vi "IRISS V2 Thorlabs.vi"() -> ()   [LabVIEW 2016]
uses:
  <vilib>/Analysis/Matrix/Datatypes/RealMatrix.ctl
  <vilib>/Math Plots/3D Math Plots/3D Scatter/3D Scatter XCtrl/3D Scatter.xctl
  Subsystems/Global Variables.vi
  <vilib>/Utility/file.llb/Read Delimited Spreadsheet (DBL).vi
  <vilib>/FPGAPlugInAG/PXI-7833R/niLvFpga_Open_PXI-7833R.vi
  <vilib>/Utility/error.llb/Error Cluster From Error Code.vi
  <vilib>/rvi/errors/niLvFpgaAdjustHostInterfaceError.vi
  <vilib>/Math Plots/3D Math Plots/3D Scatter/3D Scatter Datatype/Public/Plot Helper (Vector).vi
  Library/mjglib/var_OCTzHomeDir.vi
  <vilib>/FPGAPlugInAG/PXI-7833R/niLvFpga_Reset_PXI-7833R.vi
  <vilib>/FPGAPlugInAG/PXI-7833R/niLvFpga_Close_PXI-7833R.vi
  <vilib>/rvi/interface/nirviOpenFPGA/nirviOpenFPGA.xnode
  FPGA Bitfiles/PhantomControlPI_FPGATarget_QuadCtr2_E2412E44.lvbitx
  IRISS_FPGA_IO.vi
  <vilib>/rvi/interface/nirviReadWriteControl/nirviReadWriteControl.xnode
  <vilib>/Math Plots/3D Math Plots/3D Plot/3D Plot Datatype/3D Plot Datatype.lvclass
  <vilib>/rvi/interface/nirviMethod/nirviMethod.xnode
  <vilib>/rvi/interface/nirviCloseFPGA/nirviCloseFPGA.xnode
  <vilib>/Analysis/Matrix/NI_Matrix.lvlib
  Functions/EyeRobotDLL.dll
  Library/KevinLibraryAll/labview2011/kevLib2011.lvlib
  <vilib>/Math Plots/3D Math Plots/3D Scatter/3D Scatter Datatype/3D Scatter Datatype.lvclass
  NiFpgaLv.dll
panel:
  in  "Calib Params?":bool
  in  "Incision":bool caption="To M/S"
  out "Trajectory Cluster":T1
  in  "OCT Z PID Gains":cluster{"Kp":dbl, "Kd":dbl, "Ki":dbl}={"Kp"=0.0003, "Kd"=0.0001, "Ki"=0.01}
  out "deltaRoll":sgl
  out "deltaXYZ":sgl[](array[numeric])
  out "Online Eye Model":T2
  in  "To Regulation":bool
  out "Eye Model Cluster":T4={"X Grid"=[], "Y Grid"=[], "Za_true Surf"=[], "Iris Center"=[], "Zp_true Surf"=[], "Pinv"=[[1.0, 0.0], [0.0, 1.0]], "za_true"=5.0, "za_work"=1.0, "zp_work"=-1.0, "zp_true"=-5.0}
  out "Update Mdl & Traj":bool=TRUE
  in  "Initialize":bool caption="To M/S"
  in  "IRISS GUI":T5(tab)
  in  "U/S Power [%]":sgl min=0 max=100 step=10
  in  "Vac Cmd [mmHg]":sgl min=0 max=600 step=50
  in  "Red Round Box":u32(colorbox)=16711690
  in  "Blue Round Box":u32(colorbox)=16860
  in  "Black Round Box":u32(colorbox)
  out "Vacuum Force [mmHg]  2":i32 caption="[mmHg]"
  in  "IV Height [mmHg]":dbl=30.0 min=0.0 max=90.0 step=10.0
  in  "Irrigation":bool
  in  "Reroute Hold [sec]":dbl=10.0 caption="Hold [sec]"
  out "Next Speed":dbl=0.8 format="%#.2gx"
  out "Current Speed":dbl=0.2 format="%#_2gx"
  out "Next Depth":dbl=40.0 format="%#_g%%"
  out "Current Depth":dbl=20.0 format="%#_6g%%"
  in  "Depth Offset":dbl min=-30.0 max=70.0 step=5.0 format="%#_g%%"
  in  "Refractive Index":dbl=1.35
  in  "PO No-Fly":dbl=5.0 step=0.1 format="%#.2g"
  out "PO Cruising":dbl=5.0 format="%#.2g"
  in  "Iris Center":dbl=5.0 step=0.1 format="%#.2g"
  in  "AN Cruising":dbl=5.0 step=0.1 format="%#.2g"
  in  "AN No-Fly":dbl=5.0 step=0.1 format="%#.2g"
  in  "Iris XY Scaling":dbl[](array[numeric])=[1.0, 1.0] caption="Iris Scaling" min=0.5 max=2.0 step=0.05
  in  "Iris XY Center":dbl[](array[numeric])=[0.0, 5.0] caption="Iris Center" min=-5.0 max=5.0 step=0.25
  out "Asgn Pt Out of Bound":bool caption="Assign Pt OOB"
  out "Emergency alarm":bool
  out "Remote sender engaged":bool
  out "State changing":bool
  out "Current Run No.":u8
  out "No. of Runs":i32=5
  out "Tip out Posit":dbl[](array[numeric]) caption="Position [mm]" format="%#.3f"
  out "Tip cmd Posit":dbl[](array[numeric]) caption="Command [mm]" format="%#.3f"
  out "State Flag Array":bool[](array[boolean])
  in  "Speed Override":u16=3
  out "Timer":i32 format="%<%M:%S>t"
  in  "Assign Point [mm]":dbl[](array[numeric])=[0.0, -7.0, -6.0]
  in  "Go to Assign Pt":bool
  out "Irrigation Engaged?":bool caption="Irrigation Engaged"
  out "Robot XYZ":refnum<class "3D Plot Datatype.lvclass">[](xcontrol)
  in  "Offset":dbl[](array[numeric])
  in  "Radial Scale":dbl=0.5
  in  "Pattern":T6(ring)=enum."Centered"
  in  "Stop-and-Go":bool
  in  "SCAN_NO":string
  in  "Gen Traj":bool
  out "Trajectory OOB":bool
  out "Current System State":T7(ring)
  in  "Current Surgical Stage":T8(ring)
  in  "Tracking Mode":u16(ring) items=["Joint Mode", "XYZ Mode"]
  in  "Stage Z [mm]":dbl=100.0 min=-120.0 max=120.0 step=0.5
  in  "Stage Y [mm]":dbl=70.0 min=-120.0 max=100.0 step=0.5
  in  "Gripper":dbl
  in  "OCT Cmd Z [mm]":dbl min=-25.0 max=14.0 step=0.5
  out "Joint Out":dbl[](array[numeric])
  out "Robot Status Array":bool[](array[boolean])
  in  "L1 [deg]":dbl=-40.0
  in  "L2 [deg]":dbl=15.0
  in  "L3 [mm]":dbl=-5.0 step=0.1
  out "Status 2":bool[](array[boolean])
  in  "L4 [deg]":dbl=-10.0 step=0.1
  in  "Home":bool
  out "OCT Z out [mm]":dbl caption="OCT Out Z [mm]" format="%#.4f"
  in  "Tool Type":i32=6
  in  "Tool Offset [mm]":dbl=-50.68
  out "Grasp out":dbl format="%#.4g"
  in  "OCTz Home Dir":bool
  in  "Remote Control Source":u16(ring) caption="Remote Source" items=["None", "Surgical Console", "Joystick", "Rigid Joystick", "Zeiss PC", "MJG C++ Teleoperation", "A-Scan", "Free Joystick 2023", "Zeiss PC 2023", "MSR Zeiss Teleoperation"]
  in  "Reset Joystick":bool caption="Encoder Reset"
  out "Send Count":u64
  out "Receive Count":u64
  out "Arm ID Ind":i32
  out "Status":bool
  in  "Stage X [mm]":dbl=30.0 min=-120.0 max=120.0 step=0.5
  out "XYZ Stage out":dbl[](array[numeric])
  out "XYZ Stage cmd":dbl[](array[numeric])
  out "DH Params":cluster{"d_DH":dbl[][], "ty":dbl[][]}
  in  "Use Online Scan":bool
  in  "Process VSCAN":bool
  in  "Restart":bool
  out "Generation Error":errorcluster
  out "Model Created":bool
  in  "Eye No":i16=1 min=1 step=1
  in  "Reroute Transit Vacf":dbl=100.0
  in  "Z Rot Axis":dbl=1.0
  in  "Z Dist Thld":dbl[](array[numeric])=[3.0, 5.0] caption="Z Distance Threshould"
  in  "Vac Extremum":dbl[](array[numeric])=[68.0, 68.0] caption="Vacuum Extremum"
  in  "Max Limit [mmHg]":dbl=600.0 min=0.0 max=600.0 step=100.0
  out "Value [mmHg]":i8
  in  "Save Data":bool
  out "File Exists":bool
  out "File Path":path
  out "Elaspsed Time [s]":sgl
  in  "Data No":i16=1 min=1 step=1
  in  "Total Time":i16=90 min=1 step=1
  in  "Min PC Gap":dbl=0.1 caption="Min PC Gap [mm]" min=0.0 max=10.0 step=0.1 format="%#.3g"
  in  "Min AC Gap":dbl=0.1 caption="Min AC Gap [mm]" min=0.0 max=10.0 step=0.1 format="%#.3g"
  out "Scaling":dbl[](array[numeric])=[1.0, 1.0, 1.0] caption="S" min=0.5 max=1.5 step=0.05 format="%#_3g"
  in  "Joint Limits":dbl[][](array[numeric])=[[-68.0, -4.0], [-26.0, 52.0], [-40.0, 23.0], [-180.0, 180.0]] format="%#.3g"
  out "First Trk Pt":dbl[](array[numeric]) format="%#.3g"
  out "Error(s) Out on Program End":errorcluster
  out "L4 Waveform Graph":dbl[](graph)
  out "L3 Waveform Graph":dbl[](graph)
  out "L2 Waveform Graph":dbl[](graph)
  out "L1 Waveform Graph":dbl[](graph)
  in  "Aiming Pt":dbl[](array[numeric])=[-40.0, 11.0, 2.0, 0.0] format="%#.3g"
  in  "Engage Pt":dbl[](array[numeric])=[-40.0, 11.0, 2.0, 0.0] format="%#.3g"
  in  "Rotation":dbl[](array[numeric])=[0.0, 0.0, 0.0] caption="R [deg]" min=-15.0 max=15.0 step=0.5 format="%#_3g"
  out "Translation":dbl[](array[numeric]) caption="T [mm]" min=-3.0 max=3.0 step=0.1 format="%#_3g"
  in  "Inc Ctrl":dbl[](array[numeric])=[0.1, 0.05, 0.05] caption="Increment Control"
  in  "Depth Ctrl Array\n(% Thickness)":dbl[](array[numeric])=[40.0, 60.0, 80.0] min=10.0 max=90.0 step=5.0 format="%#_g%%"
  out "Stage command":dbl[](array[numeric])
  in  "Vscan path":path=path "D:/IRISSoft LV2016 beta/Host Demo/ThorlabsData/Eye1/VSCAN_0002.raw"
  in  "size_xyz_mm":dbl[](array[numeric])=[16.0, 16.0, 9.4, 1.0]
  in  "size_xyz":dbl[](array[numeric])=[400.0, 400.0, 1024.0, 1.0]
  in  "Confirm":bool
  in  "Image index":i32=200
  out "O":dbl[](array[numeric])
  out "New TOI":dbl[][](array[numeric])
  out "Original TOI":dbl[][](array[numeric])
  in  "Load Traj":bool caption="To M/S"
  in  "MS/Auto":bool
  in  "Retract":bool caption="To M/S"
  in  "Stop Accurus":bool caption="To M/S"
  in  "L3 Go Home":bool caption="To M/S"
  in  "Track":bool caption="To M/S"
  in  "Insert":bool caption="To M/S"
  in  "Program Stop":bool
  # "M/S\n \nAuto"
  # "Tool Tip Location"
  # "Tracking Planning"
  # "RCM"
  # "X\nY\nZ"
  # "X\nY\nZ"
  # "Tool"
  # "Trajectory"
  # "System Progress"
  # "Assign Point Rerouting"
  # "Trajectory Generation"
  # "X\nY\nZ"
  # "X Offset"
  # "Y Offset"
  # "Homing finished"
  # "Z Offset"
  # "M/S initialization finished"
  # "Tool Cruising Boundaries"
  # "XY-plane"
  # "Trajecoty loading finished"
  # "Aiming finished"
  # "Tool engaged"
  # "Z-axis"
  # "Phaco Machine"
  # "Tracking initialization finished"
  # "In Tracking"
  # "Rerouting finished"
  # "X\nY"
  # "X\nY"
  # "In regulation"
  # "Robot Control"
  # "Homing"
  # "Joint Definition"
  # "Arm"
  # "Tool"
  # "Stage"
  # "Robot Status"
  # "Joint M/S Cmd"
  # "HARDWARE_NOT_PRESENT"
  # "HARDWARE_NOT_FOUND_ALL_DRIVES"
  # "HARDWARE_SENSOR_FAULT"
  # "NOT_RUNNING"
  # "COMMUNICATION_ERROR"
  # "KINEMATICS_NO_SOLUTION"
  # "OCT Control"
  # "KINEMATICS_INSERTION_LENGTH_TOO_SMALL"
  # "COMMAND_BEYOND_JOINT_RANGE"
  # "COMMAND_TOO_LARGE"
  # "Eye Model Creation"
  # "Irrigation and Aspiration"
  # "IOP Control"
  # "Data Saving"
  # "Irrigation"
  # "Aspiration"
  # "ACh"
  # "Vitreous"
  # "Rotation & Vacuum Force Scheduling"
  # "Joint Motion & Control"
  # "Space Deform Parameters"
  # "Depth Ctrl"
  # "S"
  # "R"
  # "[deg]"
  # "T"
  # "[mm]"
  # "First Track Point"
  # "AC & PC Gap"
  # "X1"
  # "[mm]"
  # "Y"
  # "[mm]"
  # "Z"
  # "[mm]"
  # "L4"
  # "[deg]"
  # "Joint Limits"
  # "Error Message"
  # "Incision"
  # "Min."
  # "Max."
  # "L1"
  # "[deg]"
  # "L1"
  # "L2"
  # "L2"
  # "[deg]"
  # "L3"
  # "[mm]"
  # "L3"
  # "L4"
  # "[deg]"
  # "L4"
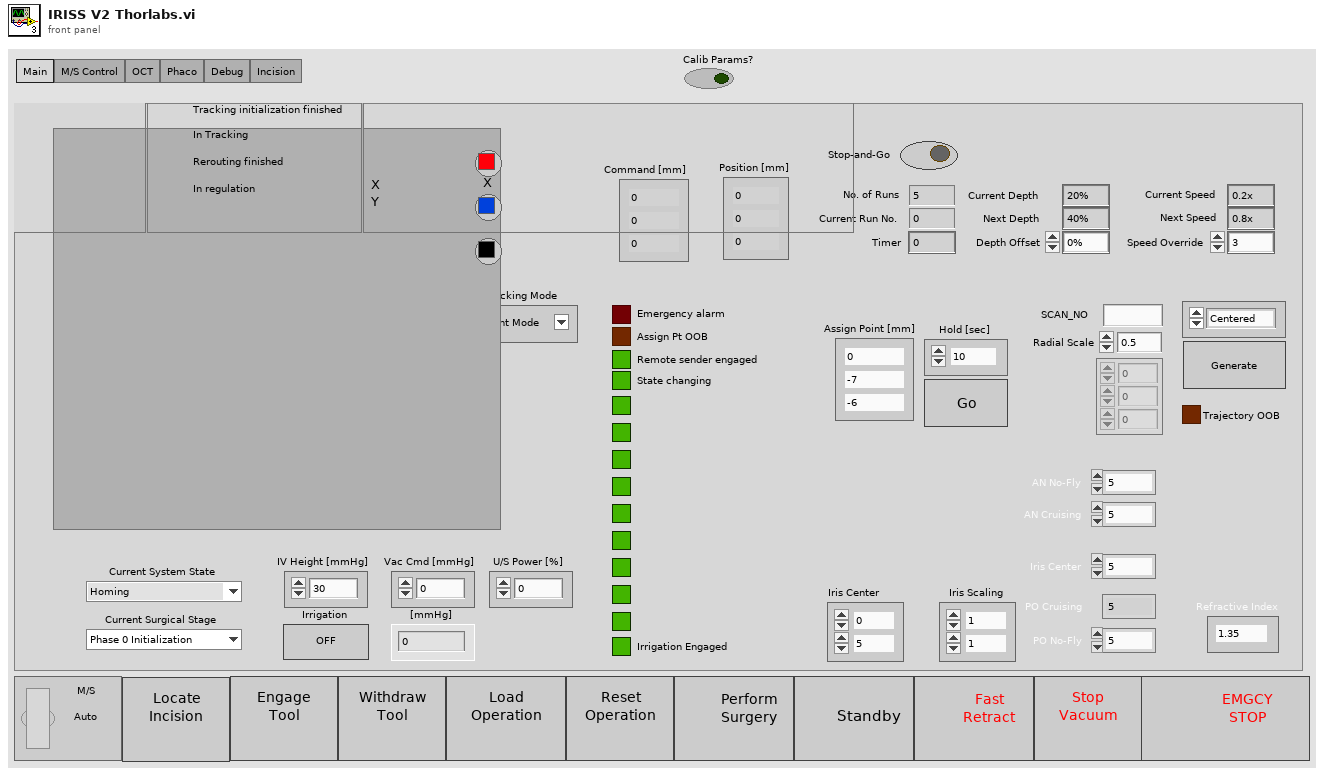
[diagram p1: front panel]
types:
  T1 = cluster{"Traj Px Array":dbl[], "Traj Py Array":dbl[], "Traj Pz Array":dbl[], "Speed Array":dbl[], "Depth Array":dbl[], "Traj Joint1 Array":dbl[], "Traj Joint2 Array":dbl[], "Traj Joint3 Array":dbl[], "Traj Joint4 Array":dbl[], "Traj Joint5 Array":dbl[]}
  T2 = cluster{"za_true":dbl, "za_work":dbl, "zi":dbl, "zp_work":dbl, "zp_true":dbl, "Iris XY Center":dbl[], "Iris XY Scaling":dbl[]}
  T3 = typedef "NI_Matrix.lvlib/RealMatrix.ctl" = dbl[][]
  T4 = cluster{"X Grid":dbl[], "Y Grid":dbl[], "Za_true Surf":dbl[][], "Iris Center":dbl[], "Zp_true Surf":dbl[][], "Pinv":T3, "za_true":dbl, "za_work":dbl, "zp_work":dbl, "zp_true":dbl}
  T5 = enum32{"Main", "M/S Control", "OCT", "Phaco", "Debug", "Incision"}
  T6 = enum16{"Entry Site", "Centered", "Insertion", "Extraction", "Reverse Entry Site", "Reverse Centered"}
  T7 = enum16{"Homing", "M/S Initialization", "M/S Operation", "Aiming", "Engaging", "Trajectory Loading", "Tracking Initialization", "Tracking", "Rerouting", "Regulation"}
  T8 = enum16{"Phase 0 Initialization", "Phase 1 Phaco", "Phase 2 Lens Removal", "Phase 3 IOL Injection"}
  T9 = enum8{"Enabled", "Disabled", "Disabled and Grayed Out"}
  T10 = cluster{"za_true_0":dbl, "za_work_0":dbl, "zp_work_0":dbl, "zp_true_0":dbl, "IrisCenter_0":dbl[]}
  T11 = cluster{"X Grid":dbl[], "Y Grid":dbl[], "Za_true Surf":dbl[][], "Iris Center":dbl[], "Zp_true Surf":dbl[][], "Real Matrix":T3, "za_true":dbl, "za_work":dbl, "zp_work":dbl, "zp_true":dbl}
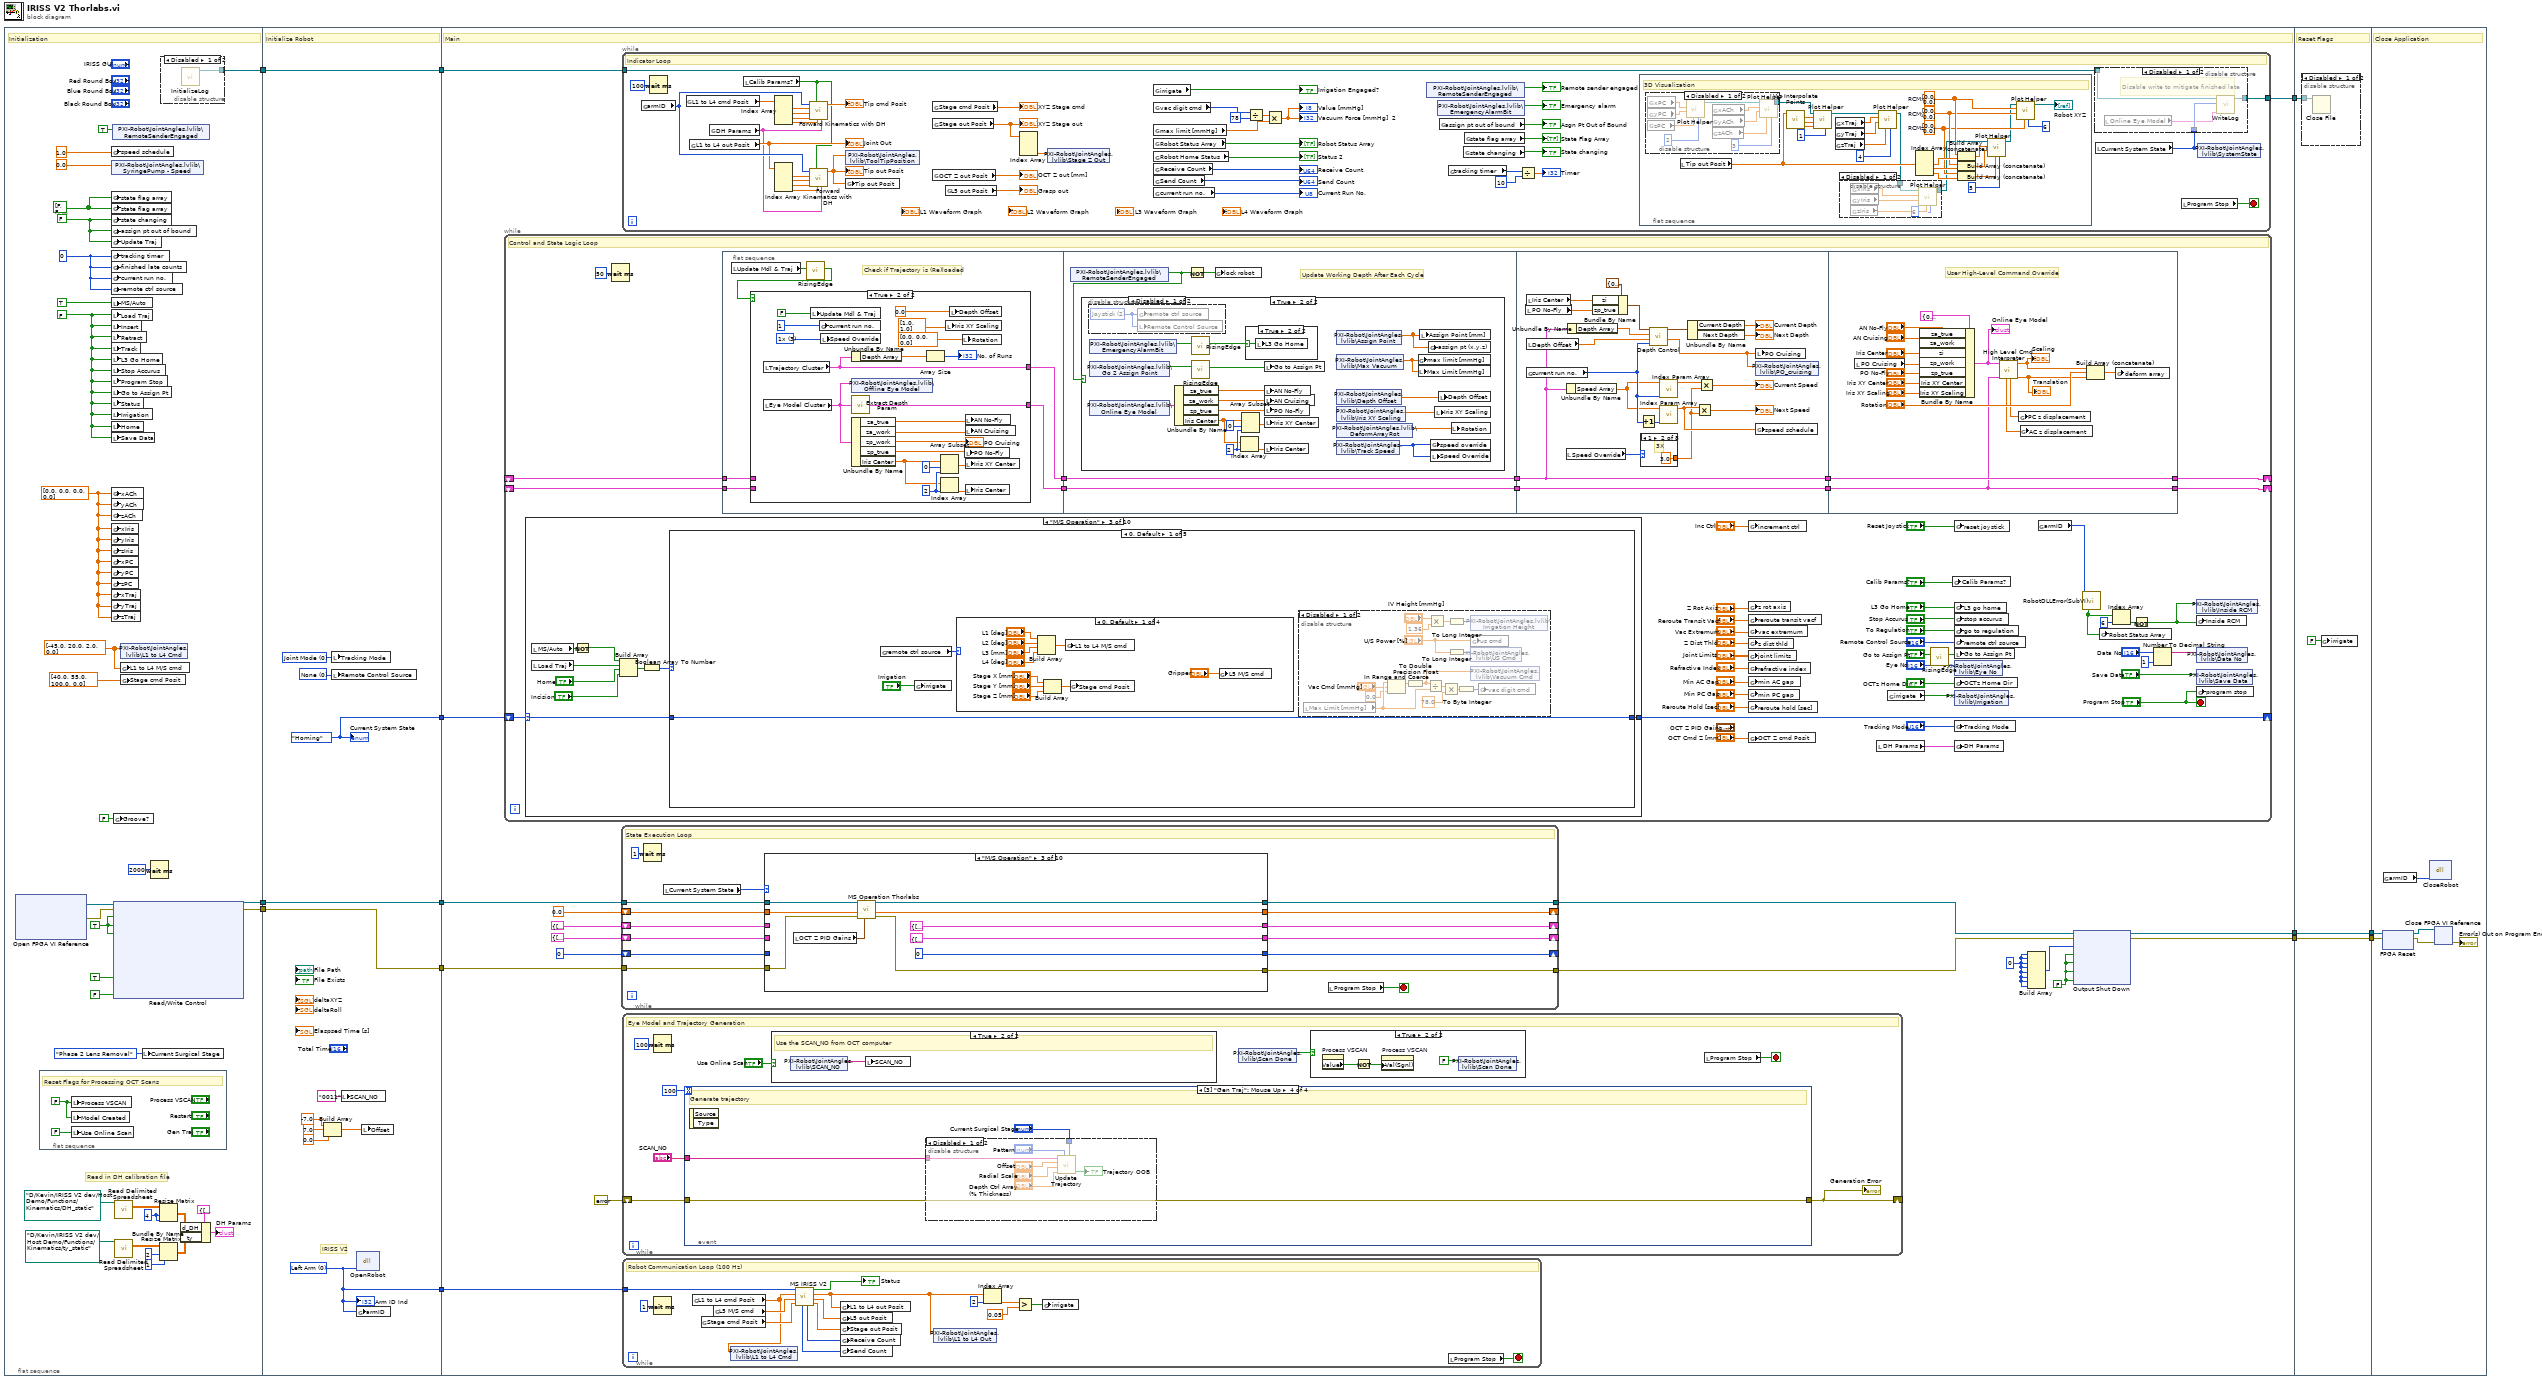
[diagram p0: block diagram]
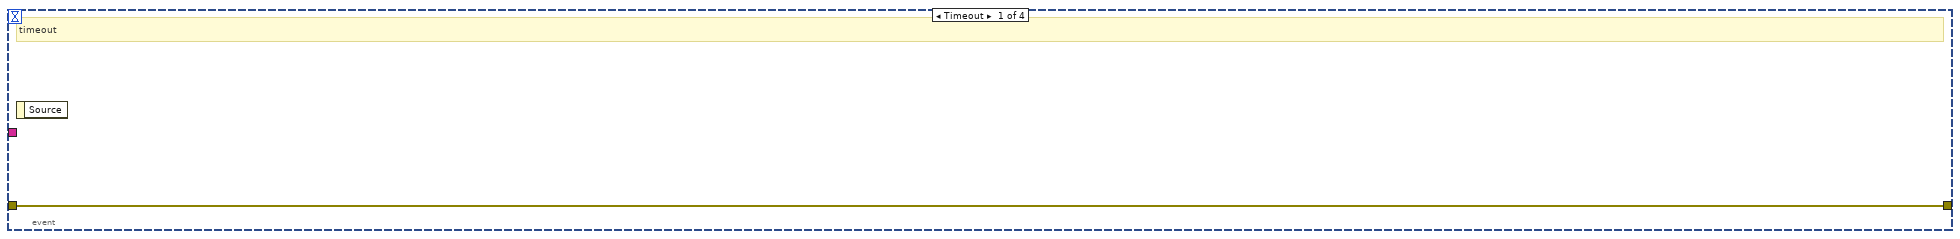
[diagram p5: hidden frame]
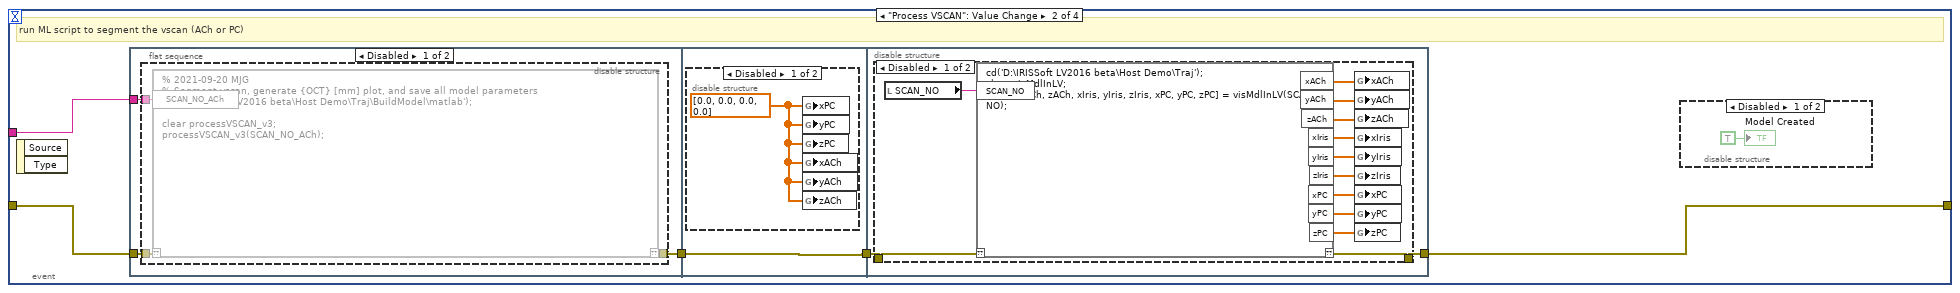
[diagram p6: hidden frame]
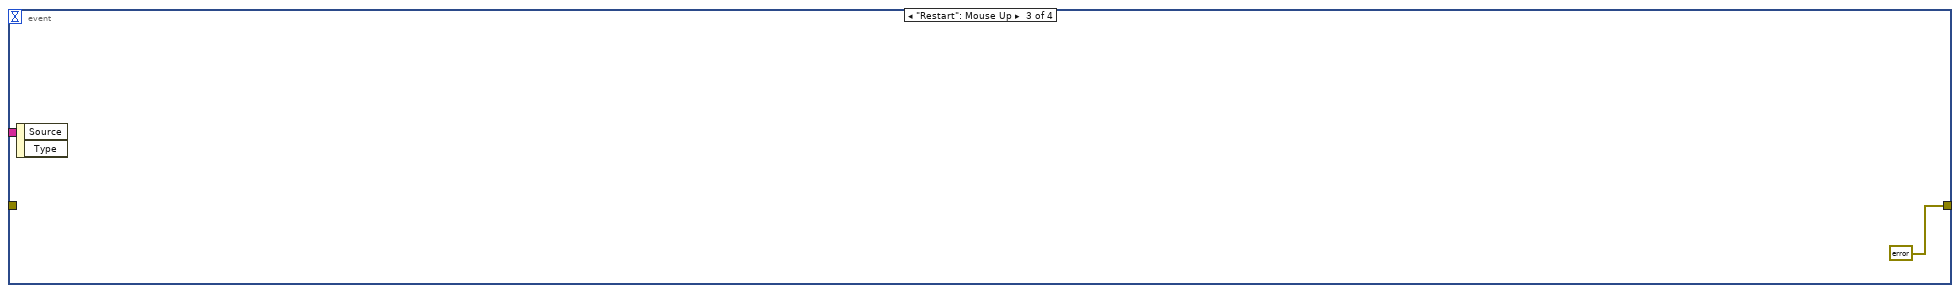
[diagram p11: hidden frame]
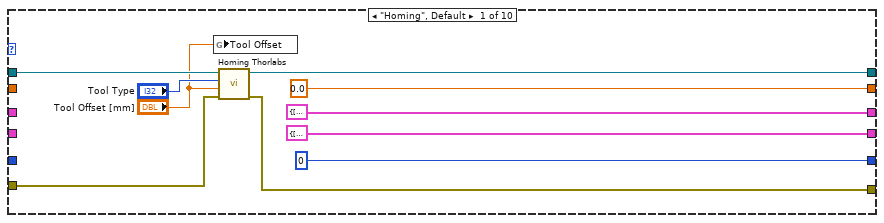
[diagram p13: hidden frame]
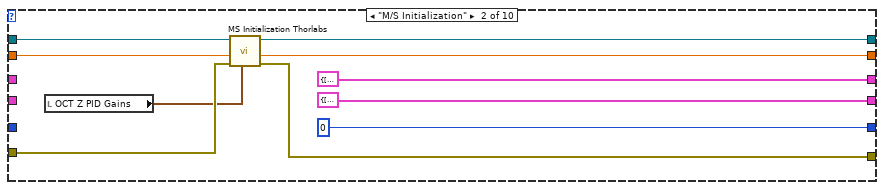
[diagram p14: hidden frame]
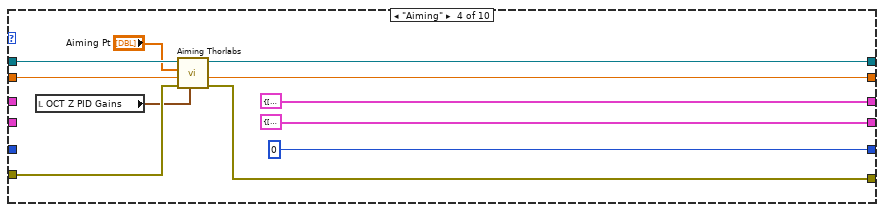
[diagram p15: hidden frame]
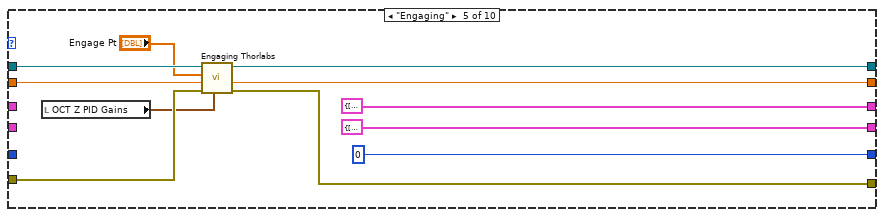
[diagram p16: hidden frame]
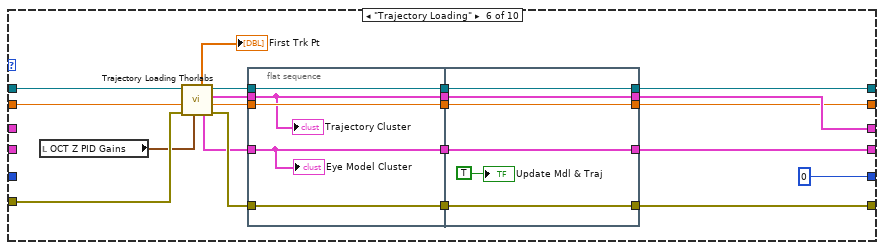
[diagram p17: hidden frame]
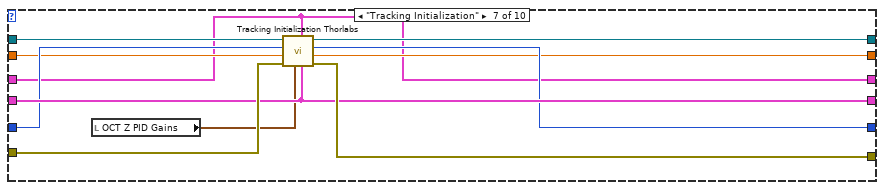
[diagram p18: hidden frame]
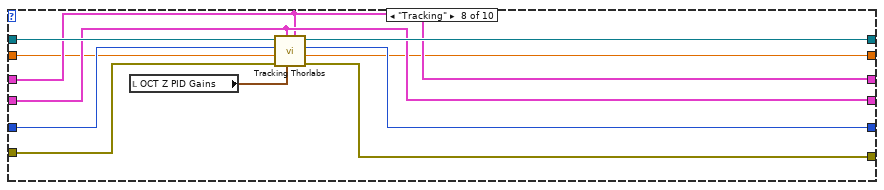
[diagram p19: hidden frame]
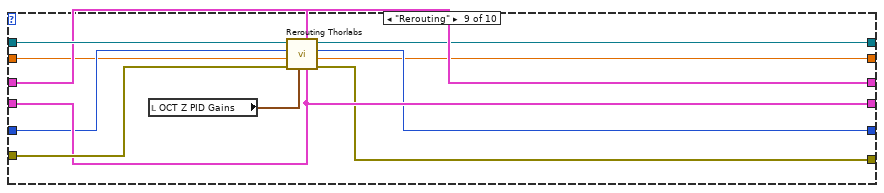
[diagram p20: hidden frame]
diagram:
  n1 = flat-sequence {
    tunnel: [w45] -> w5
    tunnel: [w37] -> w3
    tunnel: [w36] -> w2
    tunnel: [w59] -> w8
    tunnel: [w60] -> w7
    tunnel: [w58] -> w6
    tunnel: w5 -> [w61]
    tunnel: [w61] -> w4
    tunnel: w3 -> [w60]
    tunnel: w2 -> [w59]
    tunnel: [w51] -> w1
    tunnel: w8 -> [w76]
    tunnel: w7 -> [w73]
    tunnel: w6 -> [w79]
    tunnel: [w74] -> w13
    tunnel: [w75] -> w12
    tunnel: w4 -> [w78]
    tunnel: [w77] -> w11
    tunnel: w1 -> [w64]
    tunnel: w13 -> [w862]
    tunnel: w12 -> [w863]
    tunnel: w11 -> [w864]
    tunnel: [w863] -> w10
    tunnel: [w862] -> w9
    tunnel: w10 -> [w871]
    tunnel: w9 -> [w870]
    frame #0 {
      w22 = 4 ("number of rows")
      w38 = TRUE ("Conn0/DIO13 Button 2")
      w34 = dbl[] [0.0, 0.0, 0.0, 0.0] ("First Trk Pt 2")
      w29 = dbl[] [-45.0, 20.0, 2.0, 0.0] ("First Trk Pt 2")
      w33 = 0 ("finished late counts")
      w44 = bool[] [FALSE, FALSE, FALSE, FALSE, FALSE, FALSE, FALSE, FALSE, FALSE] ("state flag array")
      w42 = FALSE ("state changing")
      w35 = FALSE ("program stop")
      # "Read in DH calibration file"
      # "Initialization"
      n2 = xnode "Open FPGA VI Reference"() -> ("FPGA VI Reference Out"=w32:refnum<k20>, "error out"=w31:errorcluster)  [unwired: 2 in]
      n3 = flat-sequence {
        frame #0 {
          w47 = FALSE ("ACh Processed")
          # "Reset Flags for Processing OCT Scans"
          n4 = local write "Process VSCAN"(w47) -> ()
          n5 = local write "Model Created"(w47) -> ()
          n6 = local write "Use Online Scan"(FALSE ("Use Online Scan")) -> ()
        }
      }
      n7 = global write "Global Variables.vi" "speed schedule"(1.0 ("speed schedule")) -> ()
      n8 = shared-variable "PXI-Robot\\JointAngles.lvlib\\SyringePump - Speed"(0.0 ("SyringePump - Speed")) -> ()  [unwired: 1 in, 1 out]
      n9 = global write "Global Variables.vi" "state flag array"(w44) -> ()
      n10 = global write "Global Variables.vi" "state flag array"(w44) -> ()
      n11 = global write "Global Variables.vi" "state changing"(w42) -> ()
      n12 = global write "Global Variables.vi" "assign pt out of bound"(w42) -> ()
      n13 = global write "Global Variables.vi" "Update Traj"(w42) -> ()
      n14 = global write "Global Variables.vi" "tracking timer"(w33) -> ()
      n15 = global write "Global Variables.vi" "finished late counts"(w33) -> ()
      n16 = global write "Global Variables.vi" "current run no."(w33) -> ()
      n17 = global write "Global Variables.vi" "remote ctrl source"(w33) -> ()
      n18 = local write "MS/Auto"(TRUE ("MS/Auto")) -> ()
      n19 = local write "Load Traj"(w35) -> ()
      n20 = local write "Insert"(w35) -> ()
      n21 = local write "Retract"(w35) -> ()
      n22 = local write "Track"(w35) -> ()
      n23 = local write "L3 Go Home"(w35) -> ()
      n24 = local write "Stop Accurus"(w35) -> ()
      n25 = local write "Program Stop"(w35) -> ()
      n26 = local write "Go to Assign Pt"(w35) -> ()
      n27 = local write "Status"(w35) -> ()
      n28 = local write "Irrigation"(w35) -> ()
      n29 = local write "Home"(w35) -> ()
      n30 = local write "Save Data"(w35) -> ()
      n31 = global write "Global Variables.vi" "xACh"(w34) -> ()
      n32 = global write "Global Variables.vi" "yACh"(w34) -> ()
      n33 = global write "Global Variables.vi" "zACh"(w34) -> ()
      n34 = global write "Global Variables.vi" "xIris"(w34) -> ()
      n35 = global write "Global Variables.vi" "yIris"(w34) -> ()
      n36 = global write "Global Variables.vi" "zIris"(w34) -> ()
      n37 = global write "Global Variables.vi" "xPC"(w34) -> ()
      n38 = global write "Global Variables.vi" "yPC"(w34) -> ()
      n39 = global write "Global Variables.vi" "zPC"(w34) -> ()
      n40 = global write "Global Variables.vi" "xTraj"(w34) -> ()
      n41 = global write "Global Variables.vi" "yTraj"(w34) -> ()
      n42 = global write "Global Variables.vi" "zTraj"(w34) -> ()
      n43 = shared-variable "PXI-Robot\\JointAngles.lvlib\\RemoteSenderEngaged"(TRUE ("RemoteSenderEngaged")) -> ()  [unwired: 1 in, 1 out]
      n44 = global write "Global Variables.vi" "Groove?"(FALSE ("Groove?")) -> ()
      n45 = xnode "Read/Write Control"("FPGA VI Reference In"=w32, "error in"=w31, "Conn0/DIO12 Button 1"=w38, "Conn0/DIO13 Button 2"=w38, "Conn0/DIO15 Button 4"=w38, "Reset 14"=TRUE, "Hydration On/Off (Connector2/DIO28)"=FALSE) -> ("FPGA VI Reference Out"=w37:refnum<k20>, "error out"=w36:errorcluster)  [unwired: 3 in, 2 out]
      n46 = call-poly <vilib>:"Read Delimited Spreadsheet.vi"("file path (dialog if empty)"=path "D:/Kevin/IRISS V2 dev/Host Demo/Functions/Kinematics/DH_static" ("file path (use dialog)")) -> ("all rows"=w23:dbl[][])  [unwired: 9 in, 5 out]
      n47 = call-poly <vilib>:"Read Delimited Spreadsheet.vi"("file path (dialog if empty)"=path "D:/Kevin/IRISS V2 dev/Host Demo/Functions/Kinematics/ty_static" ("file path (use dialog)")) -> ("all rows"=w21:dbl[][])  [unwired: 9 in, 5 out]
      n48 = shared-variable "PXI-Robot\\JointAngles.lvlib\\L1 to L4 Cmd"(w29) -> ()  [unwired: 1 in, 1 out]
      n49 = global write "Global Variables.vi" "L1 to L4 M/S cmd"(w29) -> ()
      n50 = global write "Global Variables.vi" "Stage cmd Posit"(dbl[] [40.0, 55.0, 100.0, 0.0] ("First Trk Pt 2")) -> ()
      n51 = local write "Current Surgical Stage"(T8."Phase 2 Lens Removal" ("Current Surgical Stage")) -> ()
      n52 = Wait (ms)(milliseconds to wait=u32 2000) -> ()  [unwired: 1 out]
      n53 = Resize Matrix(1:w22, 2:w22, 4:w23) -> (0:w17:dbl[][])
      n54 = Resize Matrix(1:1 ("number of columns"), 2:2 ("number of rows"), 4:w21) -> (0:w16:dbl[][])
      n55 = disable-structure shown="Disabled" {
        disable-tunnel: [w49 _] -> w45
        frame Disabled {
          n56 = call "InitializeLog.vi"() -> ("Byte Stream File out"=w49:refnum<file>)  [unwired: 11 in]
        }
        frame Enabled {
        }
      }
      n57 = Bundle By Name(cluster=cluster{"d_DH":dbl[][], "ty":dbl[][]} {"d_DH"=[[0.0, -0.04858099004841317, 1.1971672750675049, 0.0], [0.0, -1.576475511297109, 0.0, 0.0], [-0.3552491783526254, 0.0, -1.1064589410656984, 0.2058446720735121], [-1.0573457532495087, 1.0278049025155533, 0.011917110633363169, -0.004023577880993236]], "ty"=[[0.04320445582455471], [0.011728642746432275]]} ("input cluster"), "d_DH"=w17, "ty"=w16) -> (→"DH Params":cluster{"d_DH":dbl[][], "ty":dbl[][]})
    }
    frame #1 {
      w50 = u16 0 items=["Joint Mode", "XYZ Mode"] ("Tracking Mode")
      w57 = u16 0 items=["None", "Surgical Console", "Joystick", "MJG Teleoperation", "MJG C++ Teleoperation"] ("Remote Control Source 2")
      w58 = T7."Homing" ("Current State")
      w51 = 0 items=["Left Arm", "Right Arm"] ("Left or Right Arm")
      # "IRISS V2"
      # "Initialize Robot"
      n58 = Build Array(-7.0 ("element"), 7.0 ("element"), 0.0 ("element")) -> (w56:dbl[])
      n59 = local write "Tracking Mode"(w50) -> ()
      n60 = local write "Remote Control Source"(w57) -> ()
      n61 = local write "SCAN_NO"("0011" ("SCAN_NO")) -> ()
      n62 = dll-call lib="D:/Kevin/IRISS V2 dev/Host Demo/Functions/EyeRobotDLL.dll" fn="OpenRobot" label="Open"("id"=w51) -> ()  [unwired: 5 in, 2 out]
      n63 = global write "Global Variables.vi" "armID"(w51) -> ()
      n64 = local write "Offset"(w56) -> ()
      "Arm ID Ind" <- w51
      "Current System State" <- w58
    }
    frame #2 {
      w67 = FALSE
      w65 = i16 0 ("element")
      # "Main"
      n65 = while {
        shift-right: [w418] -> _
        shift-left: w79 -> [w419]
        shift-right: [w415] -> _
        shift-left: _ -> [w413]
        shift-right: [w414] -> _
        shift-left: _ -> [w412]
        stop <- "Program Stop" stop-if-true
        # "Control and State Logic Loop"
        n66 = case shown="\"M/S Operation\"" w419 {
          selector: w419 -> [w533 w540 w567 w653 w673 w699 w708 w739 w783 w811]
          tunnel: [w532 w541 w566 w652 w674 w700 w709 w740 w784 w812] -> w418
          frame "Homing", Default {
            # "State Diagram"
            n67 = global read "Global Variables.vi" "state flag array"() -> (w534:bool[])
            n68 = Index Array(array=w534, index=0) -> (element=w531:bool)
            n69 = case shown="False" w531 {
              tunnel: [w536 w538] -> w532
              tunnel: w533 -> [w536 _]
              frame False {
                # "homing in process"
              }
              frame True {
                w538 = T7."M/S Initialization" ("Current State")
                # "finish homing"
                n70 = global write "Global Variables.vi" "state changing"(TRUE ("state changing")) -> ()
                n71 = global write "Global Variables.vi" "Enforce Homing"(FALSE ("Enforce Homing")) -> ()
                n72 = local write "Current System State"(w538) -> ()
              }
            }
          }
          frame "M/S Initialization" {
            n73 = global read "Global Variables.vi" "state flag array"() -> (w543:bool[])
            n74 = Index Array(array=w543, index=1) -> (element=w542:bool)
            n75 = case shown="False" w542 {
              tunnel: [w554 w556] -> w541
              tunnel: w540 -> [w554 _]
              frame False {
                n76 = global read "Global Variables.vi" "Stage cmd Posit"() -> (w548:dbl[])
                n77 = property on="MS/Auto" class="Bool (strict)"("DisabledEnum"=T9."Disabled and Grayed Out" ("Disabled")) -> ()  [unwired: 2 in, 2 out]
                n78 = Index Array(array=w548) -> (element #1=w546:dbl, element #2=w547:dbl, element #3=w545:dbl)  [unwired: 3 in]
                n79 = global read "Global Variables.vi" "L1 to L4 M/S cmd"() -> (w553:dbl[])
                n80 = local write "Stage X [mm]"(w546) -> ()
                n81 = local write "Stage Y [mm]"(w547) -> ()
                n82 = local write "Stage Z [mm]"(w545) -> ()
                n83 = Index Array(array=w553) -> (element #1=w552:dbl, element #2=w551:dbl, element #3=w550:dbl, element #4=w549:dbl)  [unwired: 4 in]
                n84 = local write "L1 [deg]"(w552) -> ()
                n85 = local write "L2 [deg]"(w551) -> ()
                n86 = local write "L3 [mm]"(w550) -> ()
                n87 = local write "L4 [deg]"(w549) -> ()
              }
              frame True {
                w556 = T7."M/S Operation" ("Current State")
                n88 = global write "Global Variables.vi" "state changing"(TRUE ("state changing")) -> ()
                n89 = property on="MS/Auto" class="Bool (strict)"("DisabledEnum"=T9."Enabled" ("Disabled")) -> ()  [unwired: 2 in, 2 out]
                n90 = local write "Current System State"(w556) -> ()
              }
            }
          }
          frame "M/S Operation" {
            n91 = local read "MS/Auto"() -> (w565:bool)
            n92 = local read "Load Traj"() -> (w563:bool)
            n93 = Not(x=w565) -> (.not. x?=w564:bool)
            n94 = Build Array(w564, w563, "Home", "Incision") -> (w562:bool[])
            n95 = Boolean Array To Number(Boolean array=w562) -> (number=w561:u32)
            n96 = case shown="0, Default" w561 {
              tunnel: w567 -> [w570 _ w610 _ w619]
              tunnel: [w570 w606 w611 w618 w619] -> w566
              frame 0, Default {
                n97 = global read "Global Variables.vi" "remote ctrl source"() -> (w569:u16)
                n98 = global write "Global Variables.vi" "irrigate"("Irrigation") -> ()
                n99 = case shown="0, Default" w569 {
                  frame 0, Default {
                    n100 = Build Array("L1 [deg]", "L2 [deg]", "L3 [mm]", "L4 [deg]") -> (w586:dbl[])
                    n101 = Build Array("Stage X [mm]", "Stage Y [mm]", "Stage Z [mm]") -> (w591:dbl[])
                    n102 = global write "Global Variables.vi" "L1 to L4 M/S cmd"(w586) -> ()
                    n103 = global write "Global Variables.vi" "Stage cmd Posit"(w591) -> ()
                    n104 = global write "Global Variables.vi" "L5 M/S cmd"("Gripper") -> ()
                  }
                  frame 1 {
                    n105 = local read "OCT Cmd Z [mm]"() -> (w596:dbl)
                    n106 = global write "Global Variables.vi" "OCT Z cmd Posit"(w596) -> ()
                  }
                  frame 2 {
                    n107 = global read "Global Variables.vi" "Stage cmd Posit"() -> (w605:dbl[])
                    n108 = Index Array(array=w605) -> (element #1=w604:dbl, element #2=w603:dbl, element #3=w602:dbl)  [unwired: 3 in]
                    n109 = local write "Stage X [mm]"(w604) -> ()
                    n110 = local write "Stage Y [mm]"(w603) -> ()
                    n111 = local write "Stage Z [mm]"(w602) -> ()
                    n112 = global read "Global Variables.vi" "L1 to L4 cmd Posit"() -> (w597:dbl[])
                    n113 = Index Array(array=w597) -> (element #1=w600:dbl, element #2=w599:dbl, element #3=w598:dbl, element #4=w601:dbl)  [unwired: 4 in]
                    n114 = local write "L1 [deg]"(w600) -> ()
                    n115 = local write "L2 [deg]"(w599) -> ()
                    n116 = local write "L3 [mm]"(w598) -> ()
                    n117 = local write "L4 [deg]"(w601) -> ()
                  }
                  frame 3 {
                  }
                }
                n118 = disable-structure shown="Disabled" {
                  frame Disabled {
                    n119 = local read "Max Limit [mmHg]"() -> (w577:dbl)
                    n120 = In Range and Coerce(upper limit=w577, x="Vac Cmd [mmHg]", lower limit=0.0) -> (coerced(x)=w578:dbl)  [unwired: 1 out]
                    n121 = To Double Precision Float(number=w578) -> (double precision float=w579:dbl)
                    n122 = Divide(x=w579, y=w577) -> (x/y=w572:dbl)
                    n123 = Multiply(x="IV Height [mmHg]", y=1.36) -> (x*y=w583:dbl)
                    n124 = Multiply(x=w572, y=78.0) -> (x*y=w574:dbl)
                    n125 = To Long Integer(number=w583) -> (32bit integer=w584:i32)
                    n126 = To Long Integer(number="U/S Power [%]") -> (32bit integer=w580:i32)
                    n127 = To Byte Integer(number=w574) -> (8bit integer=w571:i8)
                    n128 = shared-variable "PXI-Robot\\JointAngles.lvlib\\Irrigation Height"(w584) -> ()  [unwired: 1 in, 1 out]
                    n129 = global write "Global Variables.vi" "us cmd"("U/S Power [%]") -> ()
                    n130 = shared-variable "PXI-Robot\\JointAngles.lvlib\\US Cmd"(w580) -> ()  [unwired: 1 in, 1 out]
                    n131 = shared-variable "PXI-Robot\\JointAngles.lvlib\\Vacuum Cmd"(w579) -> ()  [unwired: 1 in, 1 out]
                    n132 = global write "Global Variables.vi" "vac digit cmd"(w571) -> ()
                  }
                  frame Enabled {
                  }
                }
              }
              frame 1 {
                w606 = T7."Aiming" ("Current State")
                n133 = global write "Global Variables.vi" "state changing"(TRUE ("state changing")) -> ()
                n134 = local write "Current System State"(w606) -> ()
                n135 = property on="MS/Auto" class="Bool (strict)"("DisabledEnum"=T9."Disabled and Grayed Out" ("Disabled")) -> ()  [unwired: 2 in, 2 out]
              }
              frame 2 {
                n136 = global read "Global Variables.vi" "Inside RCM"() -> (w609:bool)
                n137 = case shown="True" w609 {
                  tunnel: [w612 w613] -> w611
                  tunnel: w610 -> [w612 _]
                  frame False {
                  }
                  frame True {
                    w613 = T7."Trajectory Loading" ("Current State")
                    w614 = FALSE ("MS/Auto")
                    n138 = global write "Global Variables.vi" "state changing"(TRUE ("state changing")) -> ()
                    n139 = local write "MS/Auto"(w614) -> ()
                    n140 = local write "Load Traj"(w614) -> ()
                    n141 = local write "Current System State"(w613) -> ()
                    n142 = property on="MS/Auto" class="Bool (strict)"("DisabledEnum"=T9."Disabled and Grayed Out" ("Disabled")) -> ()  [unwired: 2 in, 2 out]
                  }
                }
              }
              frame 4 {
                w618 = T7."Homing" ("Current State")
                w617 = TRUE ("state changing")
                n143 = global write "Global Variables.vi" "state changing"(w617) -> ()
                n144 = global write "Global Variables.vi" "Enforce Homing"(w617) -> ()
                n145 = local write "Current System State"(w618) -> ()
              }
              frame 8 {
                n146 = flat-sequence {
                  frame #0 {
                    n147 = while {
                      shift-right: [w626] -> _
                      shift-left: 0 -> [w627]
                      shift-right: [w624] -> _
                      shift-left: 1 -> [w625]
                      stop <- "Confirm" stop-if-true
                      n148 = script code="if index>400\n  index_ = 400;\nelseif index<=0\n  index_ = 1;\nelse\n  index_ = index;\nend"("index"="Image index") -> ("index_"=w626:dbl)  [unwired: 1 in, 1 out]
                      n149 = Wait (ms)(milliseconds to wait=u32 100) -> ()  [unwired: 1 out]
                      n150 = Not Equal?(x=w627, y=w626) -> (x != y?=w628:bool)
                      n151 = case shown="True" w628 {
                        tunnel: w626 -> [_ w637]
                        tunnel: w625 -> [w630 w635]
                        tunnel: [w630 w634] -> w624
                        frame False {
                        }
                        frame True {
                          n152 = Path To String(path="Vscan path") -> (string=w636:string)
                          n153 = script code="%size_xyz = [400 400 1024];\nsize_xyz = size_xyz(1:3);\nframe = 1;\n% showBscanImage(filename,frame,index,size_xyz,size_xyz_mm,first_time);\nif first_time\n  fid = fopen(filename);\n  % Read the intensity values (n x 1) vector (takes some time)\n  vscan = fread(fid, prod(size_xyz), 'float32');\n  vscan = reshape(vscan, flip(size_xyz));\n\n  % nicely scale the vscan\n  vscan = vscan2nice(vscan);\n  vscan = uint8(vscan);\nend\nif frame==0\n  new_size0 = [256 int32(256*size_xyz_mm(2)/size_xyz_mm(3))];\n  img0 = filplr(imresize(vscan(:,:,index),new_size0));\n  figure(1);imshow(img0);title(['Frame:0 Index:' num2str(index)]);\nelseif frame==1\n  new_size1 = [256 int32(256*size_xyz_mm(1)/size_xyz_mm(3))];\n  temp = vscan(:,index,:);\n  img1 = reshape(temp,[size(temp,1) size(temp,3)]);\n  img1 = fliplr(imresize(img1,new_size1));\n  figure(1);imshow(img1);title(['Frame:1 Index:' num2str(index)]);\nend\n\nfirst_time = 0;"("index"=w637, "size_xyz_mm"="size_xyz_mm", "size_xyz"="size_xyz", "filename"=w636, "first_time"=w635) -> ("first_time"=w634:dbl)  [unwired: 1 in, 1 out]
                        }
                      }
                      n154 = local write "Image index"(w626) -> ()
                    }
                  }
                  frame #1 {
                    n155 = local read "size_xyz_mm"() -> (w649:dbl[])
                    n156 = local read "Image index"() -> (w650:i32)
                    n157 = local read "Vscan path"() -> (w647:path)
                    n158 = local read "size_xyz"() -> (w648:dbl[])
                    n159 = Path To String(path=w647) -> (string=w646:string)
                    n160 = script code="%size_xyz_mm = [16 16 9.4];\n%size_xyz = [400 400 1024];\nsize_xyz = size_xyz(1:3);\nframe = 1;\n%INJECTloc_OCT=IOLSEG3(filename,frame,index,size_xyz,size_xyz_mm);\n\nif frame==0\n  image = fliplr(vscan(:,:,index));\n  size_xz_mm = [size_xyz_mm(2) size_xyz_mm(3)];\n  px2mm = size_xz_mm./[size_xyz(2) size_xyz(3)]; \nelseif frame==1\n  temp = vscan(:,index,:);\n  image = fliplr(reshape(temp,[size(temp,1) size(temp,3)]));\n  size_xz_mm = [size_xyz_mm(1) size_xyz_mm(3)];\n  px2mm = size_xz_mm./[size_xyz(1) size_xyz(3)]; \nend\n%% Only to look at the center scan plan\nfigure(2); clf; \nimshow(image); hold on;\n    \n% Collect two user clicks of Injection location \n[input1, Zinput1] = ginput(1);\nplot(input1, Zinput1, 'rx', 'MarkerSize', 20, 'LineWidth', 3); \n[input2, Zinput2] = ginput(1); % Collect two user clicks \nplot(input2, Zinput2, 'rx', 'MarkerSize', 20, 'LineWidth', 3); \n    \nYinput1 = size_xyz(2) - input1; \nYinput2 = size_xyz(2) - input2;\n    \nINJECTloc_px = [Yinput1, Zinput1; ... \n        Yinput2, Zinput2]; % [px] \nINJECTloc_px_mid=[(INJECTloc_px(1,1)+INJECTloc_px(2,1))/2,(INJECTloc_px(2,1)+INJECTloc_px(2,2))/2];\nclose(2); % close figure\n    \n% Convert these two locations from pixels to {OCT} frame  \nxloc_OCT = index/400*size_xz_mm(1); % B-scan is halfway through the image\nINJECTloc_OCT = [xloc_OCT*ones(1,1), INJECTloc_px_mid(1,1)*px2mm(1),  INJECTloc_px_mid(1,2)*px2mm(2)];\n\nincision_pt = [INJECTloc_OCT(1:3),1]';\nTOI_file= 'D:\\IRISSoft LV2016 beta\\Host Demo\\TOI_static'\nfid_TOI = fopen(TOI_file,'r');\nTOI=fscanf(fid_TOI,'%f');\nTOI= reshape(TOI, [4 4])';\nfclose(fid_TOI);\n\nO = inv(TOI)*incision_pt;\n%init_X = 40;init_Y = 55;init_Z = 100;\n%time_to_go = norm(O(1:3))/.5;\n%traj = [linspace(0,O(1),1000*time_to_go);linspace(0,O(2),1000*time_to_go);linspace(0,O(3),1000*time_to_go)];\n%stage_X = linspace(init_X,init_X+O(1),1000*time_to_go);\n%stage_Y = linspace(init_Y,init_Y+O(2),1000*time_to_go);\n%stage_Z = linspace(init_Z,init_Z+O(3),1000*time_to_go);\n\nTOI2 = inv(TOI);TOI2(1:3,4) = TOI2(1:3,4)-O(1:3);\nTOI2 = inv(TOI2);\nO = O';\n\nTOI2_file= 'D:\\IRISSoft LV2016 beta\\Host Demo\\new_TOI.txt';\nfid_TOI2 = fopen(TOI2_file,'w');\nfmt = [repmat('%.10f ', 1, 4), '\\n'];\nfprintf(fid_TOI2, fmt, TOI2');\nfclose(fid_TOI2);"("index"=w650, "size_xyz_mm"=w649, "size_xyz"=w648, "filename"=w646) -> ("TOI"=→"Original TOI":dbl[][], "TOI2"=→"New TOI":dbl[][], "O"=w643:dbl[])  [unwired: 1 in, 1 out]
                    "O" <- w643
                    n161 = local read "XYZ Stage out"() -> (w642:dbl[])
                    n162 = Add(x=w643, y=w642) -> (x+y=w641:dbl[])
                    "Stage command" <- w641
                    n163 = Index Array(array=w641) -> (element #1=w640:dbl, element #2=w639:dbl, element #3=w638:dbl)  [unwired: 3 in]
                    n164 = local write "Stage X [mm]"(w640) -> ()
                    n165 = local write "Stage Y [mm]"(w639) -> ()
                    n166 = local write "Stage Z [mm]"(w638) -> ()
                  }
                  frame #2 {
                    n167 = local write "Incision"(FALSE) -> ()
                  }
                }
              }
            }
          }
          frame "Aiming" {
            n168 = global read "Global Variables.vi" "state flag array"() -> (w655:bool[])
            n169 = Index Array(array=w655, index=3) -> (element=w654:bool)
            n170 = case shown="True" w654 {
              tunnel: w653 -> [w657 w661]
              tunnel: [w657 w660] -> w652
              frame False {
              }
              frame True {
                n171 = property on="MS/Auto" class="Bool (strict)"("DisabledEnum"=T9."Enabled" ("Disabled")) -> ()  [unwired: 2 in, 2 out]
                n172 = Build Array("Insert", "MS/Auto") -> (w665:bool[])
                n173 = Boolean Array To Number(Boolean array=w665) -> (number=w662:u32)
                n174 = case shown="1" w662 {
                  tunnel: w661 -> [w666 _ _]
                  tunnel: [w666 w667 w671] -> w660
                  frame 0, Default {
                  }
                  frame 1 {
                    w667 = T7."Engaging" ("Current State")
                    n175 = global write "Global Variables.vi" "state changing"(TRUE ("state changing")) -> ()
                    n176 = local write "Insert"(FALSE ("Enter")) -> ()
                    n177 = property on="MS/Auto" class="Bool (strict)"("DisabledEnum"=T9."Disabled and Grayed Out" ("Disabled")) -> ()  [unwired: 2 in, 2 out]
                    n178 = local write "Current System State"(w667) -> ()
                  }
                  frame 2 {
                    w671 = T7."M/S Initialization" ("Current State")
                    n179 = global write "Global Variables.vi" "state changing"(TRUE ("state changing")) -> ()
                    n180 = local write "Current System State"(w671) -> ()
                  }
                }
                n181 = local read "OCT Cmd Z [mm]"() -> (w658:dbl)
                n182 = global write "Global Variables.vi" "OCT Z cmd Posit"(w658) -> ()
              }
            }
          }
          frame "Engaging" {
            n183 = global read "Global Variables.vi" "state flag array"() -> (w676:bool[])
            n184 = Index Array(array=w676, index=4) -> (element=w675:bool)
            n185 = case shown="True" w675 {
              tunnel: [w679 w686] -> w674
              tunnel: w673 -> [w680 w687]
              frame False {
                n186 = local read "Retract"() -> (w678:bool)
                n187 = case shown="False" w678 {
                  tunnel: [w681 w682] -> w679
                  tunnel: w680 -> [w681 _]
                  frame False {
                  }
                  frame True {
                    w682 = T7."Aiming" ("Current State")
                    n188 = global write "Global Variables.vi" "state changing"(TRUE ("state changing")) -> ()
                    n189 = local write "Retract"(FALSE ("Retract")) -> ()
                    n190 = local write "Current System State"(w682) -> ()
                  }
                }
              }
              frame True {
                n191 = Build Array("Load Traj", "Retract") -> (w690:bool[])
                n192 = Boolean Array To Number(Boolean array=w690) -> (number=w688:u32)
                n193 = case shown="2" w688 {
                  tunnel: w687 -> [w691 _ _]
                  tunnel: [w691 w692 w695] -> w686
                  frame 0, Default {
                  }
                  frame 1 {
                    w692 = T7."Trajectory Loading" ("Current State")
                    n194 = global write "Global Variables.vi" "state changing"(TRUE ("state changing")) -> ()
                    n195 = local write "Load Traj"(FALSE ("Load Traj")) -> ()
                    n196 = local write "Current System State"(w692) -> ()
                  }
                  frame 2 {
                    w695 = T7."Aiming" ("Current State")
                    n197 = global write "Global Variables.vi" "state changing"(TRUE ("state changing")) -> ()
                    n198 = local write "Retract"(FALSE ("Load Traj")) -> ()
                    n199 = local write "Current System State"(w695) -> ()
                  }
                }
              }
            }
          }
          frame "Trajectory Loading" {
            n200 = global read "Global Variables.vi" "state flag array"() -> (w702:bool[])
            n201 = global write "Global Variables.vi" "irrigate"(TRUE ("irrigate")) -> ()
            n202 = Index Array(array=w702, index=2) -> (element=w701:bool)
            n203 = case shown="False" w701 {
              tunnel: [w704 w705] -> w700
              tunnel: w699 -> [w704 _]
              frame False {
              }
              frame True {
                w705 = T7."Tracking Initialization" ("Current State")
                n204 = global write "Global Variables.vi" "state changing"(TRUE ("state changing")) -> ()
                n205 = local write "Current System State"(w705) -> ()
              }
            }
          }
          frame "Tracking Initialization" {
            n206 = global read "Global Variables.vi" "state flag array"() -> (w711:bool[])
            n207 = Index Array(array=w711, index=5) -> (element=w710:bool)
            n208 = case shown="True" w710 {
              tunnel: [w713 w720] -> w709
              tunnel: w708 -> [w713 w719]
              frame False {
              }
              frame True {
                n209 = local read "Load Traj"() -> (w721:bool)
                n210 = local read "Retract"() -> (w715:bool)
                n211 = local read "To Regulation"() -> (w714:bool)
                n212 = Or(x="Initialize", y=w715) -> (x .or. y?=w717:bool)
                n213 = Build Array("Track", w721, w717, w714) -> (w723:bool[])
                n214 = Boolean Array To Number(Boolean array=w723) -> (number=w722:u32)
                n215 = case shown="1" w722 {
                  tunnel: [w724 w725 w728 w731 w734] -> w720
                  tunnel: w719 -> [w724 _ _ _ _]
                  frame 0, Default {
                  }
                  frame 1 {
                    w725 = T7."Tracking" ("Current State")
                    n216 = global write "Global Variables.vi" "state changing"(TRUE ("state changing")) -> ()
                    n217 = local write "Track"(FALSE ("Track")) -> ()
                    n218 = local write "Current System State"(w725) -> ()
                  }
                  frame 2 {
                    w728 = T7."Trajectory Loading" ("Current State")
                    n219 = global write "Global Variables.vi" "state changing"(TRUE ("state changing")) -> ()
                    n220 = local write "Load Traj"(FALSE ("Load Traj")) -> ()
                    n221 = local write "Current System State"(w728) -> ()
                  }
                  frame 4 {
                    w731 = T7."Engaging" ("Current State")
                    n222 = global write "Global Variables.vi" "state changing"(TRUE ("state changing")) -> ()
                    n223 = local write "Initialize"(FALSE ("Load Traj")) -> ()
                    n224 = local write "Current System State"(w731) -> ()
                  }
                  frame 8 {
                    w734 = T7."Tracking" ("Current State")
                    w735 = FALSE  # Reset
                    n225 = global write "Global Variables.vi" "state changing"(TRUE ("state changing")) -> ()
                    n226 = local write "Track"(FALSE ("Track")) -> ()
                    n227 = local write "Current System State"(w734) -> ()
                    n228 = local write "To Regulation"(w735) -> ()
                  }
                }
              }
            }
            n229 = global write "Global Variables.vi" "irrigate"(TRUE ("irrigate")) -> ()
          }
          frame "Tracking" {
            n230 = global read "Global Variables.vi" "state flag array"() -> (w742:bool[])
            n231 = global write "Global Variables.vi" "irrigate"(TRUE ("irrigate")) -> ()
            n232 = Index Array(array=w742, index=6) -> (element=w741:bool)
            n233 = case shown="True" w741 {
              tunnel: [w744 w765] -> w740
              tunnel: w739 -> [w744 w764]
              frame False {
              }
              frame True {
                (unwired) 90 ("y")
                # "2022-08-09 Kevin\nPhaco one groove at a time"
                n234 = global read "Global Variables.vi" "Groove?"() -> (w745:bool)
                n235 = local read "Initialize"() -> (w761:bool)
                n236 = local read "Retract"() -> (w758:bool)
                n237 = local read "Go to Assign Pt"() -> (w759:bool)
                n238 = local read "To Regulation"() -> (w760:bool)
                n239 = local read "Timer"() -> (w757:i32)
                n240 = local read "Total Time"() -> (w749:i16)
                n241 = global write "Global Variables.vi" "irrigate"(TRUE ("irrigate")) -> ()
                n242 = Quotient & Remainder(x=w757, y=w749) -> (x-y*floor(x/y)=w756:i32, floor(x/y)=w752:i32)
                n243 = Equal To 0?(x=w756) -> (x = 0?=w755:bool)
                n244 = Not Equal To 0?(x=w752) -> (x != 0?=w751:bool)
                n245 = call "RisingEdge.vi"("Signal In"=w755) -> ("Rising Edge"=w754:bool)  [unwired: 10 in]
                n246 = feedback #1() -> (w747:bool)  [unwired: 1 in]
                n247 = feedback-in #1(w745) -> ()
                n248 = Compound Arithmetic op=AND(w754, w751, "Stop-and-Go") -> ()  [unwired: 1 out]
                n249 = Not Equal?(x=w745, y=w747) -> (x != y?=w746:bool)
                n250 = Build Array(w761, w758, w759, w760, FALSE ("element"), w746) -> (w763:bool[])
                n251 = Boolean Array To Number(Boolean array=w763) -> (number=w762:u32)
                n252 = case shown="32" w762 {
                  tunnel: [w766 w767 w770 w773 w776 w779 w781] -> w765
                  tunnel: w764 -> [w766 _ _ _ _ _ _]
                  frame 0, Default {
                  }
                  frame 1 {
                    w767 = T7."Engaging" ("Current State")
                    n253 = global write "Global Variables.vi" "state changing"(TRUE ("state changing")) -> ()
                    n254 = local write "Initialize"(FALSE ("Load Traj")) -> ()
                    n255 = local write "Current System State"(w767) -> ()
                  }
                  frame 2 {
                    w770 = T7."Aiming" ("Current State")
                    n256 = global write "Global Variables.vi" "state changing"(TRUE ("state changing")) -> ()
                    n257 = local write "Retract"(FALSE ("Load Traj")) -> ()
                    n258 = local write "Current System State"(w770) -> ()
                  }
                  frame 4 {
                    w773 = T7."Rerouting" ("Current State")
                    n259 = global write "Global Variables.vi" "state changing"(TRUE ("state changing")) -> ()
                    n260 = local write "Go to Assign Pt"(FALSE ("Load Traj")) -> ()
                    n261 = local write "Current System State"(w773) -> ()
                  }
                  frame 8 {
                    w776 = T7."Regulation" ("Current State")
                    n262 = global write "Global Variables.vi" "state changing"(TRUE ("state changing")) -> ()
                    n263 = local write "Current System State"(w776) -> ()
                  }
                  frame 16 {
                    w779 = T7."Regulation" ("Current State")
                    w778 = TRUE ("state changing")
                    n264 = global write "Global Variables.vi" "state changing"(w778) -> ()
                    n265 = local write "To Regulation"(w778) -> ()
                    n266 = local write "Current System State"(w779) -> ()
                  }
                  frame 32 {
                    w781 = T7."Trajectory Loading" ("Current State")
                    n267 = global write "Global Variables.vi" "state changing"(TRUE ("state changing")) -> ()
                    n268 = local write "Current System State"(w781) -> ()
                  }
                }
              }
            }
          }
          frame "Rerouting" {
            n269 = global read "Global Variables.vi" "state flag array"() -> (w786:bool[])
            n270 = Index Array(array=w786, index=7) -> (element=w785:bool)
            n271 = case shown="True" w785 {
              tunnel: [w790 w804] -> w784
              tunnel: w783 -> [w789 _]
              frame False {
                n272 = shared-variable "PXI-Robot\\JointAngles.lvlib\\EmergencyAlarmBit"() -> (w796:bool)  [unwired: 1 in, 1 out]
                n273 = local read "Initialize"() -> (w795:bool)
                n274 = local read "Retract"() -> (w788:bool)
                n275 = local read "Go to Assign Pt"() -> (w792:bool)
                n276 = Compound Arithmetic op=OR(w796, w795, w788) -> (w793:bool)
                n277 = Build Array(w793, w792) -> (w794:bool[])
                n278 = Boolean Array To Number(Boolean array=w794) -> (number=w791:u32)
                n279 = case shown="2" w791 {
                  tunnel: w789 -> [w797 _ _]
                  tunnel: [w797 w798 w801] -> w790
                  frame 0, Default {
                  }
                  frame 1 {
                    w798 = T7."Engaging" ("Current State")
                    n280 = global write "Global Variables.vi" "state changing"(TRUE ("state changing")) -> ()
                    n281 = local write "Initialize"(FALSE ("Initialize")) -> ()
                    n282 = local write "Current System State"(w798) -> ()
                  }
                  frame 2 {
                    w801 = T7."Rerouting" ("Current State")
                    n283 = global write "Global Variables.vi" "state changing"(TRUE ("state changing")) -> ()
                    n284 = local write "Go to Assign Pt"(FALSE ("Initialize")) -> ()
                    n285 = local write "Current System State"(w801) -> ()
                  }
                }
              }
              frame True {
                n286 = local read "To Regulation"() -> (w805:bool)
                n287 = case shown="False" w805 {
                  tunnel: [T7."Tracking" ("Current State") T7."Regulation" ("Current State")] -> w804
                  frame False {
                    n288 = global write "Global Variables.vi" "state changing"(TRUE ("state changing")) -> ()
                  }
                  frame True {
                    n289 = global write "Global Variables.vi" "state changing"(TRUE ("state changing")) -> ()
                  }
                }
                n290 = local write "Current System State"(w804) -> ()
              }
            }
            n291 = global write "Global Variables.vi" "irrigate"(TRUE ("irrigate")) -> ()
          }
          frame "Regulation" {
            n292 = global read "Global Variables.vi" "state flag array"() -> (w814:bool[])
            n293 = global write "Global Variables.vi" "irrigate"(TRUE ("irrigate")) -> ()
            n294 = Index Array(array=w814, index=8) -> (element=w813:bool)
            n295 = case shown="True" w813 {
              tunnel: [w823 w835] -> w812
              tunnel: w811 -> [w822 w836]
              frame False {
                n296 = local read "Initialize"() -> (w821:bool)
                n297 = local read "Retract"() -> (w820:bool)
                n298 = local read "Go to Assign Pt"() -> (w816:bool)
                n299 = Or(x=w821, y=w820) -> (x .or. y?=w819:bool)
                n300 = Build Array(w819, w816) -> (w818:bool[])
                n301 = Boolean Array To Number(Boolean array=w818) -> (number=w817:u32)
                n302 = case shown="2" w817 {
                  tunnel: w822 -> [w824 _ _]
                  tunnel: [w824 w826 w829] -> w823
                  frame 0, Default {
                  }
                  frame 1 {
                    w825 = FALSE  # Reset
                    w826 = T7."Engaging" ("Current State")
                    n303 = global write "Global Variables.vi" "state changing"(TRUE ("state changing")) -> ()
                    n304 = local write "Initialize"(FALSE ("Load Traj")) -> ()
                    n305 = local write "Current System State"(w826) -> ()
                    n306 = local write "To Regulation"(w825) -> ()
                  }
                  frame 2 {
                    w829 = T7."Rerouting" ("Current State")
                    n307 = global write "Global Variables.vi" "state changing"(TRUE ("state changing")) -> ()
                    n308 = local write "Go to Assign Pt"(FALSE ("Initialize")) -> ()
                    n309 = local write "Current System State"(w829) -> ()
                  }
                }
              }
              frame True {
                n310 = local read "Load Traj"() -> (w838:bool)
                n311 = local read "Go to Assign Pt"() -> (w839:bool)
                n312 = local read "Initialize"() -> (w834:bool)
                n313 = local read "Retract"() -> (w832:bool)
                n314 = local read "Track"() -> (w833:bool)
                n315 = Build Array(w838, w839, w834, w832, w833) -> (w840:bool[])
                n316 = Boolean Array To Number(Boolean array=w840) -> (number=w837:u32)
                n317 = case shown="8" w837 {
                  tunnel: w836 -> [w841 _ _ _ _ _]
                  tunnel: [w841 w843 w846 w850 w854 w858] -> w835
                  frame 0, Default {
                  }
                  frame 1 {
                    w842 = FALSE  # Reset
                    w843 = T7."Trajectory Loading" ("Current State")
                    n318 = global write "Global Variables.vi" "state changing"(TRUE ("state changing")) -> ()
                    n319 = local write "Load Traj"(FALSE ("Load Traj")) -> ()
                    n320 = local write "Current System State"(w843) -> ()
                    n321 = local write "To Regulation"(w842) -> ()
                  }
                  frame 2 {
                    w846 = T7."Rerouting" ("Current State")
                    n322 = global write "Global Variables.vi" "state changing"(TRUE ("state changing")) -> ()
                    n323 = local write "Go to Assign Pt"(FALSE ("Load Traj")) -> ()
                    n324 = local write "Current System State"(w846) -> ()
                  }
                  frame 4 {
                    w849 = FALSE  # Reset
                    w850 = T7."Engaging" ("Current State")
                    n325 = global write "Global Variables.vi" "state changing"(TRUE ("state changing")) -> ()
                    n326 = local write "Initialize"(FALSE ("Load Traj")) -> ()
                    n327 = local write "To Regulation"(w849) -> ()
                    n328 = local write "Current System State"(w850) -> ()
                  }
                  frame 8 {
                    w853 = FALSE  # Reset
                    w854 = T7."Aiming" ("Current State")
                    n329 = global write "Global Variables.vi" "state changing"(TRUE ("state changing")) -> ()
                    n330 = local write "Retract"(FALSE ("Load Traj")) -> ()
                    n331 = local write "To Regulation"(w853) -> ()
                    n332 = local write "Current System State"(w854) -> ()
                  }
                  frame 16 {
                    w857 = FALSE  # Reset
                    w858 = T7."Tracking" ("Current State")
                    n333 = global write "Global Variables.vi" "state changing"(TRUE ("state changing")) -> ()
                    n334 = local write "Track"(FALSE ("Load Traj")) -> ()
                    n335 = local write "Current System State"(w858) -> ()
                    n336 = local write "To Regulation"(w857) -> ()
                  }
                }
              }
            }
          }
        }
        n337 = Wait (ms)(milliseconds to wait=u32 50) -> ()  [unwired: 1 out]
        n338 = flat-sequence {
          tunnel: [w432] -> w404
          tunnel: [w431] -> w403
          tunnel: w413 -> [w430]
          tunnel: w412 -> [w429]
          tunnel: w404 -> [w460]
          tunnel: w403 -> [w459]
          tunnel: [w460] -> w402
          tunnel: [w459] -> w401
          tunnel: w402 -> [w488]
          tunnel: [w488] -> w400
          tunnel: w401 -> [w505]
          tunnel: [w505] -> w399
          tunnel: w400 -> [w528]
          tunnel: w399 -> [w518]
          tunnel: [w518] -> w414
          tunnel: [w528] -> w415
          frame #0 {
            # "Check if Trajectory is (Re)loaded"
            n339 = local read "Update Mdl & Traj"() -> (w434:bool)
            n340 = call "RisingEdge.vi"("Signal In"=w434) -> ("Rising Edge"=w433:bool)  [unwired: 10 in]
            n341 = case shown="True" w433 {
              tunnel: [w435 w456] -> w431
              tunnel: [w436 w445] -> w432
              tunnel: w430 -> [w436 _]
              tunnel: w429 -> [w435 _]
              frame False {
                # "Use Nominal Model & Trajectory"
              }
              frame True {
                w438 = u16 3 items=["4x", "3x", "2x", "1x", "0.5x", "0.2x", "0.1x", "PAUSE"] ("Speed Override")
                w450 = 2 ("index")
                # "Update Trajectory and Model after \"Trajectory Loading\""
                n342 = local read "Trajectory Cluster"() -> (w445:T1)
                n343 = local read "Eye Model Cluster"() -> (w443:T4)
                n344 = local write "Update Mdl & Traj"(FALSE ("Update Model")) -> ()
                n345 = global write "Global Variables.vi" "current run no."(u8 1 ("current run no.")) -> ()
                n346 = local write "Speed Override"(w438) -> ()
                n347 = Unbundle By Name(w445) -> ("Depth Array"=w447:dbl[])
                n348 = shared-variable "PXI-Robot\\JointAngles.lvlib\\Offline Eye Model"(w443) -> ()  [unwired: 1 in, 1 out]
                n349 = call "Extract Depth Param.vi"("Eye Model Cluster"=w443) -> ("Nominal Model param"=w456:T10)
                n350 = Unbundle By Name(w443) -> ("za_true"=w455:dbl, "za_work"=w454:dbl, "zp_work"=→"PO Cruising":dbl, "zp_true"=w452:dbl, "Iris Center"=w449:dbl[])
                n351 = Array Size(array=w447) -> (size(s)=→"No. of Runs":i32)
                n352 = Index Array(array=w449, index=w450) -> (element=w453:dbl)
                n353 = Array Subset(array=w449, index=0, length=w450) -> (w448:dbl[])
                n354 = local write "Iris XY Scaling"(dbl[] [1.0, 1.0]) -> ()
                n355 = local write "Depth Offset"(0.0 ("Depth Offset")) -> ()
                n356 = local write "Rotation"(dbl[] [0.0, 0.0, 0.0]) -> ()
                n357 = local write "PO No-Fly"(w452) -> ()
                n358 = local write "AN No-Fly"(w455) -> ()
                n359 = local write "AN Cruising"(w454) -> ()
                n360 = local write "Iris XY Center"(w448) -> ()
                n361 = local write "Iris Center"(w453) -> ()
              }
            }
          }
          frame #1 {
            # "Update Working Depth After Each Cycle"
            n362 = shared-variable "PXI-Robot\\JointAngles.lvlib\\RemoteSenderEngaged"() -> (w457:bool)  [unwired: 1 in, 1 out]
            n363 = case shown="True" w457 {
              frame False {
                n364 = global write "Global Variables.vi" "assign pt (x,y,z)"("Assign Point [mm]") -> ()
                n365 = global write "Global Variables.vi" "max limit [mmHg]"("Max Limit [mmHg]") -> ()
                n366 = global write "Global Variables.vi" "speed override"("Speed Override") -> ()
              }
              frame True {
                w468 = 2 ("index")
                n367 = disable-structure shown="Disabled" {
                  frame Disabled {
                    w483 = u16 2 items=["None", "Surgical Console", "Joystick", "MJG Teleoperation", "MJG C++ Teleoperation"] ("Remote Control Source 2")
                    n368 = global write "Global Variables.vi" "remote ctrl source"(w483) -> ()
                    n369 = local write "Remote Control Source"(w483) -> ()
                  }
                  frame Enabled {
                  }
                }
                n370 = shared-variable "PXI-Robot\\JointAngles.lvlib\\EmergencyAlarmBit"() -> (w480:bool)  [unwired: 1 in, 1 out]
                n371 = shared-variable "PXI-Robot\\JointAngles.lvlib\\Go 2 Assign Point"() -> (w477:bool)  [unwired: 1 in, 1 out]
                n372 = shared-variable "PXI-Robot\\JointAngles.lvlib\\Online Eye Model"() -> (w473:T11)  [unwired: 1 in, 1 out]
                n373 = Unbundle By Name(w473) -> ("za_true"=w476:dbl, "za_work"=w475:dbl, "zp_true"=w474:dbl, "Iris Center"=w465:dbl[])
                n374 = call "RisingEdge.vi"("Signal In"=w480) -> ("Rising Edge"=w479:bool)  [unwired: 10 in]
                n375 = call "RisingEdge.vi"("Signal In"=w477) -> ("Rising Edge"=w478:bool)  [unwired: 10 in]
                n376 = Index Array(array=w465, index=w468) -> (element=w466:dbl)
                n377 = Array Subset(array=w465, index=0, length=w468) -> (w469:dbl[])
                n378 = case shown="True" w479 {
                  selector: w479 -> [_ w484]
                  frame False {
                  }
                  frame True {
                    n379 = local write "L3 Go Home"(w484) -> ()
                  }
                }
                n380 = local write "Go to Assign Pt"(w478) -> ()
                n381 = local write "AN No-Fly"(w476) -> ()
                n382 = local write "AN Cruising"(w475) -> ()
                n383 = local write "PO No-Fly"(w474) -> ()
                n384 = local write "Iris XY Center"(w469) -> ()
                n385 = local write "Iris Center"(w466) -> ()
                n386 = shared-variable "PXI-Robot\\JointAngles.lvlib\\Assign Point"() -> (w481:dbl[])  [unwired: 1 in, 1 out]
                n387 = shared-variable "PXI-Robot\\JointAngles.lvlib\\Max Vacuum"() -> (w464:dbl)  [unwired: 1 in, 1 out]
                n388 = shared-variable "PXI-Robot\\JointAngles.lvlib\\Depth Offset"() -> (w472:dbl)  [unwired: 1 in, 1 out]
                n389 = shared-variable "PXI-Robot\\JointAngles.lvlib\\Iris XY Scaling"() -> (w471:dbl[])  [unwired: 1 in, 1 out]
                n390 = shared-variable "PXI-Robot\\JointAngles.lvlib\\DeformArrayRot"() -> (w470:dbl[])  [unwired: 1 in, 1 out]
                n391 = shared-variable "PXI-Robot\\JointAngles.lvlib\\Track Speed"() -> (w482:u16)  [unwired: 1 in, 1 out]
                n392 = global write "Global Variables.vi" "max limit [mmHg]"(w464) -> ()
                n393 = local write "Max Limit [mmHg]"(w464) -> ()
                n394 = local write "Assign Point [mm]"(w481) -> ()
                n395 = global write "Global Variables.vi" "assign pt (x,y,z)"(w481) -> ()
                n396 = global write "Global Variables.vi" "speed override"(w482) -> ()
                n397 = local write "Speed Override"(w482) -> ()
                n398 = local write "Iris XY Scaling"(w471) -> ()
                n399 = local write "Depth Offset"(w472) -> ()
                n400 = local write "Rotation"(w470) -> ()
              }
            }
            n401 = Not(x=w457) -> (.not. x?=w458:bool)
            n402 = global write "Global Variables.vi" "lock robot"(w458) -> ()
          }
          frame #2 {
            n403 = local read "PO No-Fly"() -> (w499:dbl)
            n404 = local read "Iris Center"() -> (w500:dbl)
            n405 = local read "Depth Offset"() -> (w504:dbl)
            n406 = global read "Global Variables.vi" "current run no."() -> (w497:u8)
            n407 = local read "Speed Override"() -> (w494:u16)
            n408 = Unbundle By Name(w488) -> ("Speed Array"=w496:dbl[])
            n409 = Unbundle By Name(w488) -> ("Depth Array"=w495:dbl[])
            n410 = Bundle By Name(cluster=cluster{"zi":dbl, "zp_true":dbl} {"zi"=0.0, "zp_true"=-2.5} ("z Cluster"), "zi"=w500, "zp_true"=w499) -> (w486:cluster{"zi":dbl, "zp_true":dbl})
            n411 = Increment(x=w497) -> (x+1=w498:u8)
            n412 = case shown="1" w494 {
              tunnel: [4.0 ("y") 3.0 ("y") 2.0 ("y") 1.0 ("y") 0.5 ("y") 0.2 ("y") 0.1 ("y") 0.0 ("y")] -> w491
              frame 0 {
                # "4X"
              }
              frame 1 {
                # "3X"
              }
              frame 2 {
                # "2X"
              }
              frame 3, Default {
                # "1x"
              }
              frame 4 {
                # "0.5x"
              }
              frame 5 {
                # "0.2x"
              }
              frame 6 {
                # "0.1x"
              }
              frame 7 {
                # "Pause"
              }
            }
            n413 = call "Depth Control.vi"("Current Run No."=w497, "Depth Offset"=w504, "Depth Array"=w495, "z Cluster"=w486) -> ("zp_work"=w485:dbl, "Schedule Depth & Speed"=w503:cluster{"Next Depth":dbl, "Current Depth":dbl})  [unwired: 6 in]
            n414 = call "Index Param Array.vi"("Index"=w497, "Array Input"=w496) -> ("Index Output"=w492:dbl)  [unwired: 9 in]
            n415 = call "Index Param Array.vi"("Index"=w498, "Array Input"=w496) -> ("Index Output"=w493:dbl)  [unwired: 9 in]
            n416 = Unbundle By Name(w503) -> ("Current Depth"=→"Current Depth":dbl, "Next Depth"=→"Next Depth":dbl)
            n417 = Multiply(x=w493, y=w491) -> (x*y=→"Next Speed":dbl)
            n418 = Multiply(x=w492, y=w491) -> (x*y=→"Current Speed":dbl)
            n419 = local write "PO Cruising"(w485) -> ()
            n420 = shared-variable "PXI-Robot\\JointAngles.lvlib\\PO_cruising"(w485) -> ()  [unwired: 1 in, 1 out]
            n421 = global write "Global Variables.vi" "speed schedule"(w493) -> ()
          }
          frame #3 {
            # "User High-Level Command Override"
            n422 = local read "PO Cruising"() -> (w520:dbl)
            n423 = Bundle By Name(cluster=T2 {"za_true"=0.0, "za_work"=0.0, "zi"=0.0, "zp_work"=0.0, "zp_true"=0.0, "Iris XY Center"=[0.0, 5.0], "Iris XY Scaling"=[1.0, 1.0]} ("High Level cmd"), "za_true"="AN No-Fly", "za_work"="AN Cruising", "zi"="Iris Center", "zp_work"=w520, "zp_true"="PO No-Fly", "Iris XY Center"="Iris XY Center", "Iris XY Scaling"="Iris XY Scaling") -> (w519:T2)
            "Online Eye Model" <- w519
            n424 = call "High Level Cmd Interpreter.vi"("Nominal Model param"=w518, "High Level cmd"=w519) -> ("Translation Array"=w515:dbl[], "Scaling Array"=w514:dbl[], "PC Displacement"=w516:dbl, "AC Displacement"=w517:dbl)  [unwired: 6 in]
            "Scaling" <- w514
            "Translation" <- w515
            n425 = global write "Global Variables.vi" "PC z displacement"(w516) -> ()
            n426 = global write "Global Variables.vi" "AC z displacement"(w517) -> ()
            n427 = Build Array (concatenate)(w514, "Rotation", w515) -> (w529:dbl[])
            n428 = global write "Global Variables.vi" "deform array"(w529) -> ()
          }
        }
        n429 = global write "Global Variables.vi" "increment ctrl"("Inc Ctrl") -> ()
        n430 = global write "Global Variables.vi" "z rot axis"("Z Rot Axis") -> ()
        n431 = global write "Global Variables.vi" "reroute transit vacf"("Reroute Transit Vacf") -> ()
        n432 = global write "Global Variables.vi" "vac extremum"("Vac Extremum") -> ()
        n433 = global write "Global Variables.vi" "z dist thld"("Z Dist Thld") -> ()
        n434 = global write "Global Variables.vi" "joint limits"("Joint Limits") -> ()
        n435 = global write "Global Variables.vi" "refractive index"("Refractive Index") -> ()
        n436 = global write "Global Variables.vi" "min AC gap"("Min AC Gap") -> ()
        n437 = global write "Global Variables.vi" "min PC gap"("Min PC Gap") -> ()
        n438 = global write "Global Variables.vi" "reroute hold [sec]"("Reroute Hold [sec]") -> ()
        n439 = global write "Global Variables.vi" "OCT Z cmd Posit"("OCT Cmd Z [mm]") -> ()
        n440 = local read "DH Params"() -> (w383:cluster{"d_DH":dbl[][], "ty":dbl[][]})
        n441 = global read "Global Variables.vi" "irrigate"() -> (w391:bool)
        n442 = call "RisingEdge.vi"("Signal In"="Go to Assign Pt") -> ("Rising Edge"=w405:bool)  [unwired: 10 in]
        n443 = global write "Global Variables.vi" "Calib Params?"("Calib Params?") -> ()
        n444 = global write "Global Variables.vi" "reset joystick"("Reset Joystick") -> ()
        n445 = global write "Global Variables.vi" "L3 go home"("L3 Go Home") -> ()
        n446 = global write "Global Variables.vi" "stop accurus"("Stop Accurus") -> ()
        n447 = global write "Global Variables.vi" "go to regulation"("To Regulation") -> ()
        n448 = global write "Global Variables.vi" "remote ctrl source"("Remote Control Source") -> ()
        n449 = local write "Go to Assign Pt"(w405) -> ()
        n450 = shared-variable "PXI-Robot\\JointAngles.lvlib\\Eye No"("Eye No") -> ()  [unwired: 1 in, 1 out]
        n451 = global write "var_OCTzHomeDir.vi" "OCTz Home Dir"("OCTz Home Dir") -> ()
        n452 = shared-variable "PXI-Robot\\JointAngles.lvlib\\Irrigation"(w391) -> ()  [unwired: 1 in, 1 out]
        n453 = global write "Global Variables.vi" "Tracking Mode"("Tracking Mode") -> ()
        n454 = global write "Global Variables.vi" "DH Params"(w383) -> ()
        n455 = global read "Global Variables.vi" "armID"() -> (w397:i32)
        n456 = call "RobotDLLError(SubVI).vi"("ArmID"=w397) -> ("RobotStatusArray"=w396:bool[])  [unwired: 5 in, 9 out]
        n457 = global write "Global Variables.vi" "Robot Status Array"(w396) -> ()
        n458 = Index Array(array=w396, index=6) -> (element=w394:bool)
        n459 = Not(x=w394) -> (.not. x?=w393:bool)
        n460 = Number To Decimal String(number="Data No", width (-)=i16 1) -> (decimal integer string=w386:string)
        n461 = shared-variable "PXI-Robot\\JointAngles.lvlib\\Inside RCM"(w393) -> ()  [unwired: 1 in, 1 out]
        n462 = global write "Global Variables.vi" "Inside RCM"(w393) -> ()
        n463 = shared-variable "PXI-Robot\\JointAngles.lvlib\\Data No"(w386) -> ()  [unwired: 1 in, 1 out]
        n464 = shared-variable "PXI-Robot\\JointAngles.lvlib\\Save Data"("Save Data") -> ()  [unwired: 1 in, 1 out]
        n465 = global write "Global Variables.vi" "program stop"("Program Stop") -> ()
      }
      n466 = while {
        tunnel: w73 -> [w161]
        tunnel: w76 -> [w160]
        tunnel: [w159] -> w69
        tunnel: [w158] -> w68
        shift-right: [w156] -> _
        shift-left: 0.0 ("Prev OCT Z Posit") -> [w157]
        shift-right: [w154] -> _
        shift-left: 0 -> [w153]
        shift-right: [w152] -> _
        shift-left: T1 {"Traj Px Array"=[], "Traj Py Array"=[], "Traj Pz Array"=[], "Speed Array"=[], "Depth Array"=[], "Traj Joint1 Array"=[], "Traj Joint2 Array"=[], "Traj Joint3 Array"=[], "Traj Joint4 Array"=[], "Traj Joint5 Array"=[]} ("Trajectory Cluster 2") -> [w150]
        shift-right: [w151] -> _
        shift-left: T4 {"X Grid"=[], "Y Grid"=[], "Za_true Surf"=[], "Iris Center"=[0.0, 5.0, 0.0], "Zp_true Surf"=[], "Pinv"=[[1.0, 0.0], [0.0, 1.0]], "za_true"=0.0, "za_work"=0.0, "zp_work"=0.0, "zp_true"=0.0} ("Eye Model Cluster") -> [w149]
        stop <- w155 stop-if-true
        # "State Execution Loop"
        n467 = Wait (ms)(milliseconds to wait=u32 1) -> ()  [unwired: 1 out]
        n468 = local read "Current System State"() -> (w148:T7)
        n469 = case shown="\"M/S Operation\"" w148 {
          tunnel: w161 -> [w170 w180 w190 w198 w210 w226 w256 w268 w279 w286]
          tunnel: w160 -> [w166 w177 w188 w201 w212 w223 w255 w267 w276 w285]
          tunnel: [w169 w179 w189 w199 w209 w233 w257 w265 w277 w287] -> w159
          tunnel: [w165 w178 w187 w200 w211 w234 w254 w266 w270 w284] -> w158
          tunnel: w157 -> [_ w176 w186 w196 w207 w222 w250 w260 w272 w282]
          tunnel: [0.0 ("Prev OCT Z Posit") w175 w185 w195 w206 w215 w249 w259 w271 w281] -> w156
          tunnel: [0 ("Last Index") 0 ("Last Index") 0 ("Last Index") 0 ("Last Index") 0 ("Last Index") 0 w251 w261 w273 w290] -> w154
          tunnel: w153 -> [_ _ _ _ _ _ w252 w262 w274 w290]
          tunnel: [T1 {"Traj Px Array"=[], "Traj Py Array"=[], "Traj Pz Array"=[], "Speed Array"=[], "Depth Array"=[], "Traj Joint1 Array"=[], "Traj Joint2 Array"=[], "Traj Joint3 Array"=[], "Traj Joint4 Array"=[], "Traj Joint5 Array"=[]} ("Trajectory Cluster 2") T1 {"Traj Px Array"=[], "Traj Py Array"=[], "Traj Pz Array"=[], "Speed Array"=[], "Depth Array"=[], "Traj Joint1 Array"=[], "Traj Joint2 Array"=[], "Traj Joint3 Array"=[], "Traj Joint4 Array"=[], "Traj Joint5 Array"=[]} ("Trajectory Cluster 2") T1 {"Traj Px Array"=[], "Traj Py Array"=[], "Traj Pz Array"=[], "Speed Array"=[], "Depth Array"=[], "Traj Joint1 Array"=[], "Traj Joint2 Array"=[], "Traj Joint3 Array"=[], "Traj Joint4 Array"=[], "Traj Joint5 Array"=[]} ("Trajectory Cluster 2") T1 {"Traj Px Array"=[], "Traj Py Array"=[], "Traj Pz Array"=[], "Speed Array"=[], "Depth Array"=[], "Traj Joint1 Array"=[], "Traj Joint2 Array"=[], "Traj Joint3 Array"=[], "Traj Joint4 Array"=[], "Traj Joint5 Array"=[]} ("Trajectory Cluster 2") T1 {"Traj Px Array"=[], "Traj Py Array"=[], "Traj Pz Array"=[], "Speed Array"=[], "Depth Array"=[], "Traj Joint1 Array"=[], "Traj Joint2 Array"=[], "Traj Joint3 Array"=[], "Traj Joint4 Array"=[], "Traj Joint5 Array"=[]} ("Trajectory Cluster 2") w232 w247 w263 w278 w289] -> w152
          tunnel: [T4 {"X Grid"=[], "Y Grid"=[], "Za_true Surf"=[], "Iris Center"=[0.0, 5.0, 0.0], "Zp_true Surf"=[], "Pinv"=[[1.0, 0.0], [0.0, 1.0]], "za_true"=0.0, "za_work"=0.0, "zp_work"=0.0, "zp_true"=0.0} ("Eye Model Cluster") T4 {"X Grid"=[], "Y Grid"=[], "Za_true Surf"=[], "Iris Center"=[0.0, 5.0, 0.0], "Zp_true Surf"=[], "Pinv"=[[1.0, 0.0], [0.0, 1.0]], "za_true"=0.0, "za_work"=0.0, "zp_work"=0.0, "zp_true"=0.0} ("Eye Model Cluster") T4 {"X Grid"=[], "Y Grid"=[], "Za_true Surf"=[], "Iris Center"=[0.0, 5.0, 0.0], "Zp_true Surf"=[], "Pinv"=[[1.0, 0.0], [0.0, 1.0]], "za_true"=0.0, "za_work"=0.0, "zp_work"=0.0, "zp_true"=0.0} ("Eye Model Cluster") T4 {"X Grid"=[], "Y Grid"=[], "Za_true Surf"=[], "Iris Center"=[0.0, 5.0, 0.0], "Zp_true Surf"=[], "Pinv"=[[1.0, 0.0], [0.0, 1.0]], "za_true"=0.0, "za_work"=0.0, "zp_work"=0.0, "zp_true"=0.0} ("Eye Model Cluster") T4 {"X Grid"=[], "Y Grid"=[], "Za_true Surf"=[], "Iris Center"=[0.0, 5.0, 0.0], "Zp_true Surf"=[], "Pinv"=[[1.0, 0.0], [0.0, 1.0]], "za_true"=0.0, "za_work"=0.0, "zp_work"=0.0, "zp_true"=0.0} ("Eye Model Cluster") w231 w253 w264 w275 w288] -> w151
          tunnel: w150 -> [_ _ _ _ _ _ w247 w263 w278 w289]
          tunnel: w149 -> [_ _ _ _ _ _ w253 w264 w275 w288]
          frame "Homing", Default {
            n470 = global write "Global Variables.vi" "Tool Offset"("Tool Offset [mm]") -> ()
            n471 = call "Homing Thorlabs.vi"("error in"=w166, "Tool Offset"="Tool Offset [mm]", "ToolType"="Tool Type", "FPGA VI Reference In"=w170) -> ("error out"=w165:errorcluster, "FPGA VI Reference Out"=w169:refnum<k20>)  [unwired: 6 in]
          }
          frame "M/S Initialization" {
            n472 = local read "OCT Z PID Gains"() -> (w174:cluster{"Kp":dbl, "Kd":dbl, "Ki":dbl})
            n473 = call "MS Initialization Thorlabs.vi"("OCT Z PID Gains"=w174, "error in"=w177, "OCT Prev Posit"=w176, "FPGA VI Reference In"=w180) -> ("error out"=w178:errorcluster, "OCT Last Posit"=w175:dbl, "FPGA VI Reference Out"=w179:refnum<k20>)  [unwired: 5 in]
          }
          frame "M/S Operation" {
            n474 = local read "OCT Z PID Gains"() -> (w184:cluster{"Kp":dbl, "Kd":dbl, "Ki":dbl})
            n475 = call "MS Operation Thorlabs.vi"("OCT Z PID Gains"=w184, "error in"=w188, "OCT Prev Posit"=w186, "FPGA VI Reference In"=w190) -> ("error out"=w187:errorcluster, "OCT Last Posit"=w185:dbl, "FPGA VI Reference Out"=w189:refnum<k20>)  [unwired: 5 in]
          }
          frame "Aiming" {
            n476 = local read "OCT Z PID Gains"() -> (w194:cluster{"Kp":dbl, "Kd":dbl, "Ki":dbl})
            n477 = call "Aiming Thorlabs.vi"("OCT Z PID Gains"=w194, "error in"=w201, "OCT Prev Posit"=w196, "Aiming Pt"="Aiming Pt", "FPGA VI Reference In"=w198) -> ("error out"=w200:errorcluster, "OCT Last Posit"=w195:dbl, "FPGA VI Reference Out"=w199:refnum<k20>)  [unwired: 4 in]
          }
          frame "Engaging" {
            n478 = local read "OCT Z PID Gains"() -> (w205:cluster{"Kp":dbl, "Kd":dbl, "Ki":dbl})
            n479 = call "Engaging Thorlabs.vi"("OCT Z PID Gains"=w205, "error in"=w212, "OCT Prev Posit"=w207, "Engage Pt"="Engage Pt", "FPGA VI Reference In"=w210) -> ("error out"=w211:errorcluster, "OCT Last Posit"=w206:dbl, "FPGA VI Reference Out"=w209:refnum<k20>)  [unwired: 4 in]
          }
          frame "Trajectory Loading" {
            n480 = local read "OCT Z PID Gains"() -> (w221:cluster{"Kp":dbl, "Kd":dbl, "Ki":dbl})
            n481 = call "Trajectory Loading Thorlabs.vi"("OCT Z PID Gains"=w221, "error in"=w223, "OCT Prev Posit"=w222, "FPGA VI Reference In"=w226) -> ("error out"=w220:errorcluster, "OCT Last Posit"=w217:dbl, "Trajectory Cluster"=w219:T1, "FPGA VI Reference Out"=w224:refnum<k20>, "Eye Model Cluster"=w218:T4, "First Trk Pt"=→"First Trk Pt":dbl[])  [unwired: 2 in]
            n482 = flat-sequence {
              tunnel: w218 -> [w238]
              tunnel: w220 -> [w240]
              tunnel: [w240] -> w230
              tunnel: w224 -> [w239]
              tunnel: [w239] -> w229
              tunnel: [w236] -> w228
              tunnel: w219 -> [w236]
              tunnel: [w238] -> w227
              tunnel: w217 -> [w237]
              tunnel: [w237] -> w216
              tunnel: [w245] -> w234
              tunnel: w230 -> [w245]
              tunnel: w229 -> [w244]
              tunnel: [w244] -> w233
              tunnel: w228 -> [w243]
              tunnel: w227 -> [w242]
              tunnel: [w243] -> w232
              tunnel: [w242] -> w231
              tunnel: w216 -> [w241]
              tunnel: [w241] -> w215
              frame #0 {
                "Eye Model Cluster" <- w238
                "Trajectory Cluster" <- w236
              }
              frame #1 {
                "Update Mdl & Traj" <- TRUE
              }
            }
          }
          frame "Tracking Initialization" {
            n483 = local read "OCT Z PID Gains"() -> (w248:cluster{"Kp":dbl, "Kd":dbl, "Ki":dbl})
            n484 = call "Tracking Initialization Thorlabs.vi"("Eye Model Cluster"=w253, "Trajectory Cluster"=w247, "OCT Z PID Gains"=w248, "error in"=w255, "OCT Prev Posit"=w250, "Prev Index"=w252, "FPGA VI Reference In"=w256) -> ("error out"=w254:errorcluster, "OCT Last Posit"=w249:dbl, "Last Index"=w251:i32, "FPGA VI Reference Out"=w257:refnum<k20>)  [unwired: 1 in]
          }
          frame "Tracking" {
            n485 = local read "OCT Z PID Gains"() -> (w258:cluster{"Kp":dbl, "Kd":dbl, "Ki":dbl})
            n486 = call "Tracking Thorlabs.vi"("Trajectory Cluster"=w263, "OCT Z PID Gains"=w258, "Eye Model Cluster"=w264, "error in"=w267, "OCT Prev Posit"=w260, "Resume Index"=w262, "FPGA VI Reference In"=w268) -> ("error out"=w266:errorcluster, "OCT Last Posit"=w259:dbl, "Leave Index"=w261:i32, "FPGA VI Reference Out"=w265:refnum<k20>)  [unwired: 1 in]
          }
          frame "Rerouting" {
            n487 = local read "OCT Z PID Gains"() -> (w269:cluster{"Kp":dbl, "Kd":dbl, "Ki":dbl})
            n488 = call "Rerouting Thorlabs.vi"("Eye Model Cluster"=w275, "Trajectory Cluster"=w278, "OCT Z PID Gains"=w269, "error in"=w276, "OCT Prev Posit"=w272, "Prev Index"=w274, "FPGA VI Reference In"=w279) -> ("error out"=w270:errorcluster, "OCT Last Posit"=w271:dbl, "Last Index"=w273:i32, "FPGA VI Reference Out"=w277:refnum<k20>)  [unwired: 1 in]
          }
          frame "Regulation" {
            n489 = local read "OCT Z PID Gains"() -> (w280:cluster{"Kp":dbl, "Kd":dbl, "Ki":dbl})
            n490 = local read "Engage Pt"() -> (w283:dbl[])
            n491 = call "Regulation Thorlabs.vi"("OCT Z PID Gains"=w280, "error in"=w285, "OCT Prev Posit"=w282, "Engage Pt"=w283, "FPGA VI Reference In"=w286) -> ("error out"=w284:errorcluster, "OCT Last Posit"=w281:dbl, "FPGA VI Reference Out"=w287:refnum<k20>)  [unwired: 4 in]
          }
        }
        n492 = local read "Program Stop"() -> (w155:bool)
      }
      n493 = while {
        tunnel: w78 -> [w324]
        tunnel: [w323] -> w77
        stop <- w333 stop-if-true
        # "Indicator Loop"
        n494 = global read "Global Variables.vi" "armID"() -> (w300:i32)
        n495 = Wait (ms)(milliseconds to wait=u32 100) -> ()  [unwired: 1 out]
        n496 = global read "Global Variables.vi" "L1 to L4 cmd Posit"() -> (w305:dbl[])
        n497 = global read "Global Variables.vi" "L1 to L4 out Posit"() -> (w299:dbl[])
        "Joint Out" <- w299
        n498 = global read "Global Variables.vi" "DH Params"() -> (w294:cluster{"d_DH":dbl[][], "ty":dbl[][]})
        n499 = local read "Calib Params?"() -> (w291:bool)
        n500 = Index Array(array=w305) -> (element #1=w304:dbl, element #2=w303:dbl, element #3=w302:dbl, element #4=w301:dbl)  [unwired: 4 in]
        n501 = Index Array(array=w299) -> (element #1=w298:dbl, element #2=w297:dbl, element #3=w296:dbl, element #4=w295:dbl)  [unwired: 4 in]
        n502 = call "Forward Kinematics with DH.vi"("DH Params"=w294, "j4"=w301, "DH Calib?"=w291, "j3"=w302, "j2"=w303, "j1"=w304, "armID"=w300) -> ("XYZ"=→"Tip cmd Posit":dbl[])  [unwired: 2 in, 2 out]
        n503 = call "Forward Kinematics with DH.vi"("DH Params"=w294, "j4"=w295, "DH Calib?"=w291, "j3"=w296, "j2"=w297, "j1"=w298, "armID"=w300) -> ("XYZ"=w292:dbl[])  [unwired: 2 in, 2 out]
        "Tip out Posit" <- w292
        n504 = shared-variable "PXI-Robot\\JointAngles.lvlib\\ToolTipPosition"(w292) -> ()  [unwired: 1 in, 1 out]
        n505 = global write "Global Variables.vi" "Tip out Posit"(w292) -> ()
        n506 = global read "Global Variables.vi" "Stage cmd Posit"() -> (→"XYZ Stage cmd":dbl[])
        n507 = global read "Global Variables.vi" "Stage out Posit"() -> (w308:dbl[])
        "XYZ Stage out" <- w308
        n508 = global read "Global Variables.vi" "OCT Z out Posit"() -> (→"OCT Z out [mm]":dbl)
        n509 = global read "Global Variables.vi" "L5 out Posit"() -> (→"Grasp out":dbl)
        n510 = Index Array(array=w308) -> (element #3=w309:dbl)  [unwired: 3 in, 2 out]
        n511 = shared-variable "PXI-Robot\\JointAngles.lvlib\\Stage Z Out"(w309) -> ()  [unwired: 1 in, 1 out]
        n512 = global read "Global Variables.vi" "irrigate"() -> (→"Irrigation Engaged?":bool)
        n513 = global read "Global Variables.vi" "vac digit cmd"() -> (w314:i8)
        n514 = global read "Global Variables.vi" "max limit [mmHg]"() -> (w311:dbl)
        n515 = global read "Global Variables.vi" "Robot Status Array"() -> (→"Robot Status Array":bool[])
        n516 = global read "Global Variables.vi" "Robot Home Status"() -> (→"Status 2":bool[])
        n517 = global read "Global Variables.vi" "Receive Count"() -> (→"Receive Count":u64)
        n518 = global read "Global Variables.vi" "Send Count"() -> (→"Send Count":u64)
        n519 = global read "Global Variables.vi" "current run no."() -> (→"Current Run No.":u8)
        n520 = Divide(x=w314, y=i8 78) -> (x/y=w312:dbl)
        n521 = Multiply(x=w312, y=w311) -> (x*y=→"Value [mmHg]" →"Vacuum Force [mmHg]  2":dbl)
        n522 = shared-variable "PXI-Robot\\JointAngles.lvlib\\RemoteSenderEngaged"() -> (→"Remote sender engaged":bool)  [unwired: 1 in, 1 out]
        n523 = shared-variable "PXI-Robot\\JointAngles.lvlib\\EmergencyAlarmBit"() -> (→"Emergency alarm":bool)  [unwired: 1 in, 1 out]
        n524 = global read "Global Variables.vi" "assign pt out of bound"() -> (→"Asgn Pt Out of Bound":bool)
        n525 = global read "Global Variables.vi" "tracking timer"() -> (w326:i32)
        n526 = global read "Global Variables.vi" "state changing"() -> (→"State changing":bool)
        n527 = global read "Global Variables.vi" "state flag array"() -> (→"State Flag Array":bool[])
        n528 = Divide(x=w326, y=10) -> (x/y=→"Timer":dbl)
        n529 = flat-sequence {
          frame #0 {
            w355 = sgl[] [0.0, 0.0]  # RCMy
            w354 = sgl[] [0.0, 0.0]  # RCMz
            w356 = sgl[] [0.0, 0.0]  # RCMx
            # "3D Visualization"
            n530 = disable-structure shown="Disabled" {
              disable-tunnel: [w365 _] -> w344
              frame Disabled {
                n531 = global read "Global Variables.vi" "xPC"() -> (w363:dbl[])
                n532 = global read "Global Variables.vi" "yPC"() -> (w362:dbl[])
                n533 = global read "Global Variables.vi" "zPC"() -> (w361:dbl[])
                n534 = call-poly <vilib>:"Plot Helper.vi"("Plot ID"=2, "z vector"=w361, "y vector"=w362, "x vector"=w363) -> ("3D Plot lvclass Array out"=w370:refnum<class "3D Plot Datatype.lvclass">[])  [unwired: 2 in, 5 out]
                n535 = global read "Global Variables.vi" "xACh"() -> (w368:dbl[])
                n536 = global read "Global Variables.vi" "yACh"() -> (w367:dbl[])
                n537 = global read "Global Variables.vi" "zACh"() -> (w366:dbl[])
                n538 = call-poly <vilib>:"Plot Helper.vi"("Plot ID"=3, "z vector"=w366, "y vector"=w367, "x vector"=w368, "3D Plot lvclass Array in"=w370) -> ("3D Plot lvclass Array out"=w365:refnum<class "3D Plot Datatype.lvclass">[])  [unwired: 1 in, 5 out]
              }
              frame Enabled {
              }
            }
            n539 = local read "Tip out Posit"() -> (w348:dbl[])
            n540 = call "Vis Interpolate Points.vi"("Tip out Posit"=w348) -> ("Z"=w345:dbl[], "Y"=w346:dbl[], "X"=w347:dbl[])  [unwired: 4 in]
            n541 = call-poly <vilib>:"Plot Helper.vi"("Plot ID"=1, "z vector"=w345, "y vector"=w346, "x vector"=w347, "3D Plot lvclass Array in"=w344) -> ("3D Plot lvclass Array out"=w338:refnum<class "3D Plot Datatype.lvclass">[])  [unwired: 1 in, 5 out]
            n542 = global read "Global Variables.vi" "xTraj"() -> (w339:dbl[])
            n543 = global read "Global Variables.vi" "yTraj"() -> (w340:dbl[])
            n544 = global read "Global Variables.vi" "zTraj"() -> (w341:dbl[])
            n545 = call-poly <vilib>:"Plot Helper.vi"("Plot ID"=4, "z vector"=w341, "y vector"=w340, "x vector"=w339, "3D Plot lvclass Array in"=w338) -> ("3D Plot lvclass Array out"=w336:refnum<class "3D Plot Datatype.lvclass">[])  [unwired: 1 in, 5 out]
            n546 = disable-structure shown="Disabled" {
              disable-tunnel: w336 -> [w372 w377]
              disable-tunnel: [w371 w377] -> w335
              frame Disabled {
                n547 = global read "Global Variables.vi" "xIris"() -> (w376:dbl[])
                n548 = global read "Global Variables.vi" "yIris"() -> (w375:dbl[])
                n549 = global read "Global Variables.vi" "zIris"() -> (w374:dbl[])
                n550 = call-poly <vilib>:"Plot Helper.vi"("Plot ID"=6, "z vector"=w374, "y vector"=w375, "x vector"=w376, "3D Plot lvclass Array in"=w372) -> ("3D Plot lvclass Array out"=w371:refnum<class "3D Plot Datatype.lvclass">[])  [unwired: 1 in, 5 out]
              }
              frame Enabled {
              }
            }
            n551 = Index Array(array=w348) -> (element #1=w359:dbl, element #2=w358:dbl, element #3=w357:dbl)  [unwired: 3 in]
            n552 = Build Array (concatenate)(w356, w359) -> (w351:dbl[])
            n553 = Build Array (concatenate)(w355, w358) -> (w350:dbl[])
            n554 = Build Array (concatenate)(w354, w357) -> (w349:dbl[])
            n555 = call-poly <vilib>:"Plot Helper.vi"("Plot ID"=5, "z vector"=w349, "y vector"=w350, "x vector"=w351, "3D Plot lvclass Array in"=w335) -> ("3D Plot lvclass Array out"=w342:refnum<class "3D Plot Datatype.lvclass">[])  [unwired: 1 in, 5 out]
            n556 = call-poly <vilib>:"Plot Helper.vi"("Plot ID"=6, "z vector"=w354, "y vector"=w355, "x vector"=w356, "3D Plot lvclass Array in"=w342) -> ("3D Plot lvclass Array out"=→"Robot XYZ":refnum<class "3D Plot Datatype.lvclass">[])  [unwired: 1 in, 5 out]
          }
        }
        n557 = local read "Current System State"() -> (w322:T7)
        n558 = disable-structure shown="Disabled" {
          disable-tunnel: w324 -> [w381 _]
          disable-tunnel: [w380 _] -> w323
          disable-tunnel: w322 -> [w379 _]
          frame Disabled {
            # "Disable write to mitigate finished late"
            n559 = local read "Online Eye Model"() -> (w378:T2)
            n560 = call "WriteLog.vi"("Online Eye Model"=w378, "Current System State"=w379, "File In"=w381) -> ("File Out"=w380:refnum<file>)  [unwired: 8 in]
          }
          frame Enabled {
          }
        }
        n561 = local read "Program Stop"() -> (w333:bool)
        n562 = shared-variable "PXI-Robot\\JointAngles.lvlib\\SystemState"(w322) -> ()  [unwired: 1 in, 1 out]
      }
      n563 = while {
        shift-right: [w97] -> _
        shift-left: errorcluster {"status"=FALSE, "code"=0, "source"=""} ("error IO") -> [w102]
        stop <- w100 stop-if-true
        # "Eye Model and Trajectory Generation"
        n564 = Wait (ms)(milliseconds to wait=u32 100) -> ()  [unwired: 1 out]
        n565 = event shown="[3] \"Gen Traj\": Mouse Up" {
          selector: _ -> [_ _ _ _]
          dyn-events: _ -> [_ _ _ _]
          timeout: 100 -> [_ _ _ _]
          tunnel: [w108 w109 errorcluster {"status"=FALSE, "code"=0, "source"=""} ("error IO") w140] -> w97
          tunnel: w102 -> [w108 w112 _ w140]
          tunnel: "SCAN_NO" -> [_ w113 _ w139]
          event Timeout {
            # "timeout"
            n566 = event-data() -> ()  [unwired: 1 in, 1 out]
          }
          event "Process VSCAN": Value Change {
            # "run ML script to segment the vscan (ACh or PC)"
            n567 = event-data() -> ()  [unwired: 1 in, 2 out]
            n568 = flat-sequence {
              tunnel: w113 -> [w117]
              tunnel: w112 -> [w116]
              tunnel: [w115] -> w111
              tunnel: w111 -> [w121]
              tunnel: [w121] -> w110
              tunnel: w110 -> [w124]
              tunnel: [w123] -> w109
              frame #0 {
                n569 = disable-structure shown="Disabled" {
                  disable-tunnel: w117 -> [w120 _]
                  disable-tunnel: w116 -> [w119 _]
                  disable-tunnel: [w118 _] -> w115
                  frame Disabled {
                    n570 = script code="% 2021-09-20 MJG \n% Segment vscan, generate {OCT} [mm] plot, and save all model parameters\ncd('D:\\IRISSoft LV2016 beta\\Host Demo\\Traj\\BuildModel\\matlab');\n\nclear processVSCAN_v3;\nprocessVSCAN_v3(SCAN_NO_ACh);"("??"=w119, "SCAN_NO_ACh"=w120) -> ("??"=w118:errorcluster)
                  }
                  frame Enabled {
                  }
                }
              }
              frame #1 {
                n571 = disable-structure shown="Disabled" {
                  frame Disabled {
                    w122 = dbl[] [0.0, 0.0, 0.0, 0.0] ("First Trk Pt 2")
                    n572 = global write "Global Variables.vi" "xPC"(w122) -> ()
                    n573 = global write "Global Variables.vi" "yPC"(w122) -> ()
                    n574 = global write "Global Variables.vi" "zPC"(w122) -> ()
                    n575 = global write "Global Variables.vi" "xACh"(w122) -> ()
                    n576 = global write "Global Variables.vi" "yACh"(w122) -> ()
                    n577 = global write "Global Variables.vi" "zACh"(w122) -> ()
                  }
                  frame Enabled {
                  }
                }
              }
              frame #2 {
                n578 = disable-structure shown="Disabled" {
                  disable-tunnel: w124 -> [w129 _]
                  disable-tunnel: [w128 _] -> w123
                  frame Disabled {
                    n579 = local read "SCAN_NO"() -> (w133:string)
                    n580 = script code="cd('D:\\IRISSoft LV2016 beta\\Host Demo\\Traj');\nclear visMdlInLV;\n[xACh, yACh, zACh, xIris, yIris, zIris, xPC, yPC, zPC] = visMdlInLV(SCAN_NO);"("??"=w129, "SCAN_NO"=w133) -> ("??"=w128:errorcluster, "xACh"=w134:dbl[], "yACh"=w135:dbl[], "zACh"=w136:dbl[], "xPC"=w132:dbl[], "yPC"=w131:dbl[], "zPC"=w130:dbl[], "xIris"=w127:dbl[], "yIris"=w126:dbl[], "zIris"=w125:dbl[])
                    n581 = global write "Global Variables.vi" "xACh"(w134) -> ()
                    n582 = global write "Global Variables.vi" "yACh"(w135) -> ()
                    n583 = global write "Global Variables.vi" "zACh"(w136) -> ()
                    n584 = global write "Global Variables.vi" "xIris"(w127) -> ()
                    n585 = global write "Global Variables.vi" "yIris"(w126) -> ()
                    n586 = global write "Global Variables.vi" "zIris"(w125) -> ()
                    n587 = global write "Global Variables.vi" "xPC"(w132) -> ()
                    n588 = global write "Global Variables.vi" "yPC"(w131) -> ()
                    n589 = global write "Global Variables.vi" "zPC"(w130) -> ()
                  }
                  frame Enabled {
                  }
                }
              }
            }
            n590 = disable-structure shown="Disabled" {
              frame Disabled {
                "Model Created" <- TRUE ("Model Created")
              }
              frame Enabled {
              }
            }
          }
          event "Restart": Mouse Up {
            n591 = event-data() -> ()  [unwired: 1 in, 2 out]
          }
          event "Gen Traj": Mouse Up {
            # "Generate trajectory"
            n592 = event-data() -> ()  [unwired: 1 in, 2 out]
            n593 = disable-structure shown="Disabled" {
              disable-tunnel: w139 -> [w147 _]
              disable-tunnel: "Current Surgical Stage" -> [w141 _]
              frame Disabled {
                n594 = call "Update Trajectory.vi"("Current Surgical Stage"=w141, "Pattern"="Pattern", "Depth Ctrl Array\n(% Thickness)"="Depth Ctrl Array\n(% Thickness)", "Scale"="Radial Scale", "Offset"="Offset", "SCAN_NO"=w147) -> ("Trajectory OOB"=→"Trajectory OOB":bool)  [unwired: 5 in]
              }
              frame Enabled {
              }
            }
          }
        }
        "Generation Error" <- w97
        n595 = case shown="True" "Use Online Scan" {
          frame False {
            # "User specified SCAN_NO"
          }
          frame True {
            # "Use the SCAN_NO from OCT computer"
            n596 = shared-variable "PXI-Robot\\JointAngles.lvlib\\SCAN_NO"() -> (w107:string)  [unwired: 1 in, 1 out]
            n597 = local write "SCAN_NO"(w107) -> ()
          }
        }
        n598 = shared-variable "PXI-Robot\\JointAngles.lvlib\\Scan Done"() -> (w98:bool)  [unwired: 1 in, 1 out]
        n599 = case shown="True" w98 {
          frame False {
          }
          frame True {
            n600 = property on="Process VSCAN" class="Bool (strict)"() -> ("Value"=w106:bool)  [unwired: 2 in, 2 out]
            n601 = Not(x=w106) -> (.not. x?=w105:bool)
            n602 = property on="Process VSCAN" class="Bool (strict)"("Val(Sgnl)"=w105) -> ()  [unwired: 2 in, 2 out]
            n603 = shared-variable "PXI-Robot\\JointAngles.lvlib\\Scan Done"(FALSE ("Scan Done")) -> ()  [unwired: 1 in, 1 out]
          }
        }
        n604 = local read "Program Stop"() -> (w100:bool)
      }
      n605 = while {
        tunnel: w64 -> [w93]
        stop <- w94 stop-if-true
        # "Robot Communication Loop (100 Hz)"
        n606 = Wait (ms)(milliseconds to wait=u32 1) -> ()  [unwired: 1 out]
        n607 = global read "Global Variables.vi" "L1 to L4 cmd Posit"() -> (w80:dbl[])
        n608 = global read "Global Variables.vi" "Stage cmd Posit"() -> (w89:dbl[])
        n609 = global read "Global Variables.vi" "L5 M/S cmd"() -> (w82:dbl)
        n610 = shared-variable "PXI-Robot\\JointAngles.lvlib\\L1 to L4 Cmd"(w80) -> ()  [unwired: 1 in, 1 out]
        n611 = call "MS IRISS V2.vi"("Stage Cmd Posit"=w89, "L5 cmd Posit"=w82, "Joint Cmd Posit"=w80, "ArmID"=w93) -> ("Stage Out Posit"=w88:dbl[], "L5 Out Posit"=w83:dbl, "Joint Out Posit"=w81:dbl[], "Connection Status"=→"Status":bool, "Receive Count"=w90:u64, "Send Count"=w91:u64)  [unwired: 2 in]
        n612 = global write "Global Variables.vi" "L1 to L4 out Posit"(w81) -> ()
        n613 = global write "Global Variables.vi" "L5 out Posit"(w83) -> ()
        n614 = global write "Global Variables.vi" "Stage out Posit"(w88) -> ()
        n615 = global write "Global Variables.vi" "Receive Count"(w90) -> ()
        n616 = global write "Global Variables.vi" "Send Count"(w91) -> ()
        n617 = shared-variable "PXI-Robot\\JointAngles.lvlib\\L1 to L4 Out"(w81) -> ()  [unwired: 1 in, 1 out]
        n618 = Index Array(array=w81, index=2) -> (element=w86:dbl)
        n619 = Greater?(x=w86, y=0.05) -> (0:w85:bool)
        n620 = global write "Global Variables.vi" "irrigate"(w85) -> ()
        n621 = local read "Program Stop"() -> (w94:bool)
      }
      n622 = Build Array(w65, w65, w65, w65, w65, w65, w65, w65) -> (w66:i16[])
      n623 = xnode "Output Shut Down"("FPGA VI Reference In"=w69, "error in"=w68, "AO"=w66, "INHB X"=w67, "INHB Y"=w67, "INHB Z"=w67, "INHB OCT Mot"=w67) -> ("FPGA VI Reference Out"=w75:refnum<k20>, "error out"=w74:errorcluster)
    }
    frame #3 {
      # "Reset Flags"
      n624 = disable-structure shown="Disabled" {
        disable-tunnel: w864 -> [w865 _]
        frame Disabled {
          n625 = Close File(refnum=w865) -> ()  [unwired: 1 in, 2 out]
        }
        frame Enabled {
        }
      }
      n626 = global write "Global Variables.vi" "irrigate"(FALSE ("irrigate")) -> ()
    }
    frame #4 {
      # "Close Application"
      n627 = xnode "FPGA Reset"("FPGA VI Reference In"=w871, "error in"=w870) -> ("FPGA VI Reference Out"=w866:refnum<k20>, "error out"=w867:errorcluster)
      n628 = global read "Global Variables.vi" "armID"() -> (w869:i32)
      n629 = dll-call lib="D:/Kevin/IRISS V2 dev/Host Demo/Functions/EyeRobotDLL.dll" fn="CloseRobot" label="Close"("id"=w869) -> ()  [unwired: 5 in, 2 out]
      n630 = xnode "Close FPGA VI Reference"("FPGA VI Reference In"=w866, "error in"=w867) -> ("error out"=→"Error(s) Out on Program End":errorcluster)
    }
  }
